vi "Batched Execution Engine.vi"() -> ()   [LabVIEW 2010]
uses:
  <vilib>/addons/database/NI_Database_API.lvlib
  <vilib>/addons/database/_DB Variant To Data/Database Variant To Data.xnode
  <vilib>/addons/database/Connection.llb/DB Tools Open Connec (String).vi
  <vilib>/xml/NI_XML.lvlib
  <vilib>/Utility/VariantDataType/VariantType.lvlib
  <vilib>/addons/database/Connection.llb/Conn Execute.vi
  <vilib>/addons/database/Recordset.llb/Rec Destroy - Connection.vi
  <vilib>/Utility/config.llb/NI_LVConfig.lvlib
  <vilib>/Utility/config.llb/Read Key (String).vi
panel:
  in  "Number of Parameters":i32
  out "Parameters Array Size":i32
  out "submit_time":timestamp
  out "exec_time":timestamp
  in  "Parameter out":T1(array[cluster])
  out "error in (no error)":errorcluster
  out "exp_id":i32
  out "Result: XML Footer":string
  out "Result: XML Header":string
  out "Control TAG":string
  out "Indicator TAG":string
  out "Experiment VI":string
  out "Database":string
  out "CSG 2":csg caption="CSG"
  out "CDB 2":cdb caption="CDB"
  out "CXT 2":cxt caption="CXT"
  out "U 65":u64 caption="U 64"
  out "U 33":u32 caption="U 32"
  out "U 17":u16 caption="U 16"
  out "I 9":i64 caption="I 8"
  out "I 65":i64 caption="I 64"
  out "EXT 2":ext caption="EXT"
  out "I16 2":i16
  out "FXP 2":fxp<+,1,1> caption="FXP"
  out "Single 2":sgl
  out "I 33":i32 caption="I 32"
  out "U 9":i32 caption="U 8"
  out "String 2":string caption="String"
  out "Double 2":dbl caption="Double"
  in  "Parameter in":cluster{"parameter":string, "datatype":string}[](array[cluster])
  out "XML-String-out":string
  in  "input array":variant[](array[variant])
  out "output array":variant[](array[variant])
  out "parse errors":string
  in  "Root in":string="/experimentSpecification/terminal/function/"
  in  "Write Status to Log file":bool
  out "XML-String-in":string
  in  "Stop":bool
  out "Status":string
  # "Parameter Tag"
  # "Parameter data type"
  # "Result Tag"
  # "Result Attribute"
  # "Settings"
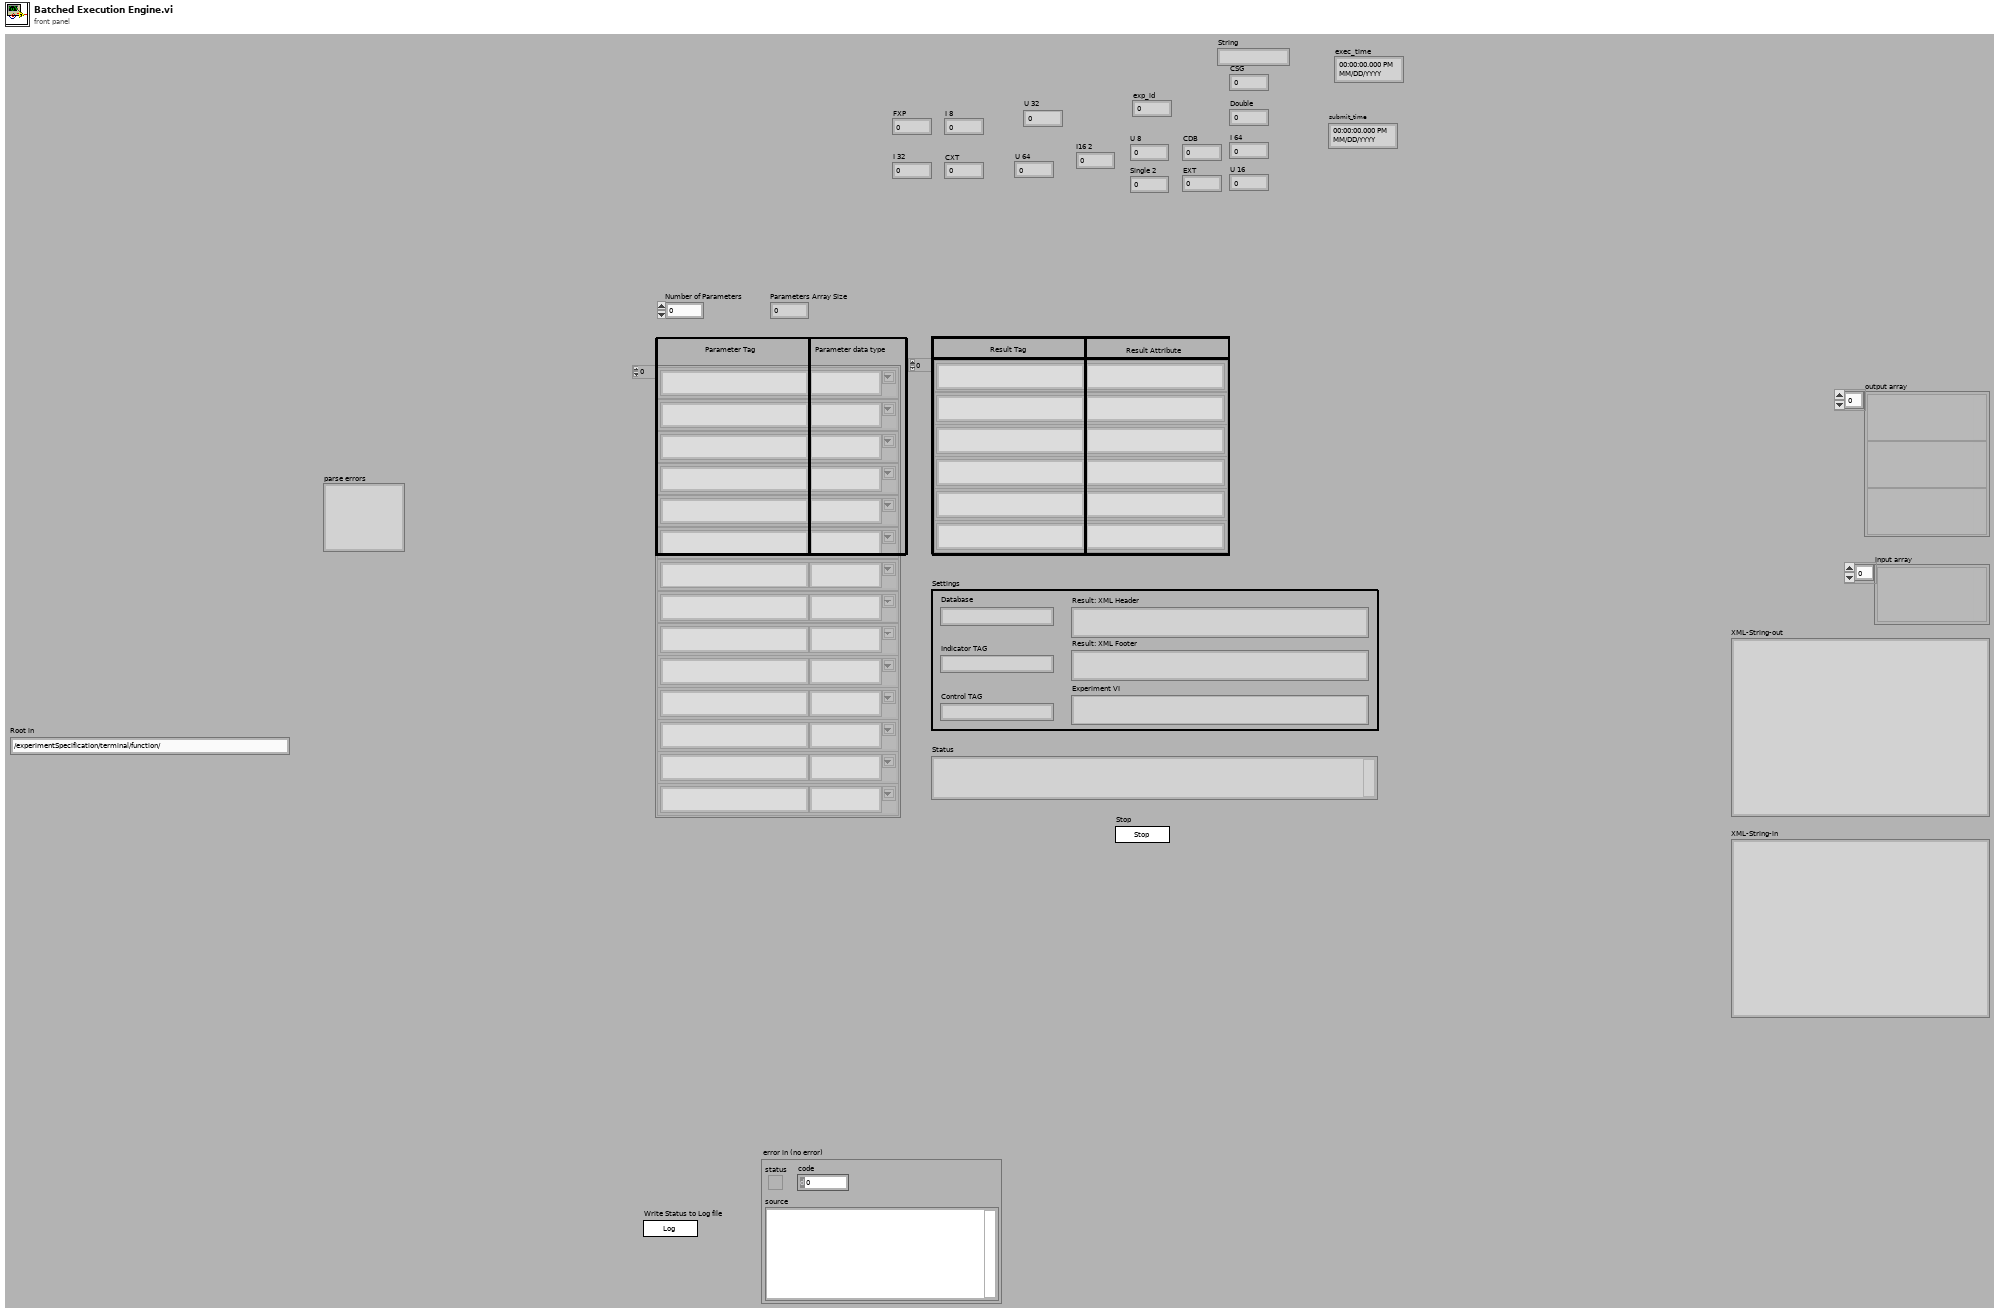
[diagram p1: front panel]
types:
  T1 = cluster{"parameter":string, "type info":string}[]
  T2 = enum16{"Search", "Parse", "Run", "Assemble", "Set", ""}
  T3 = typedef "NI_LVConfig.lvlib/Config Data RefNum.ctl" = refnum<k1>
  T4 = typedef "NI_Database_API.lvlib/Conn ObjectReference.ctl" = refnum<k1>
  T5 = typedef "NI_Database_API.lvlib/Rec ObjectReference.ctl" = refnum<k1>
  T6 = typedef "VariantType.lvlib/Type.ctl" = enum8{"Invalid Type", "Void", "I8", "I16", "I32", "I64", "U8", "U16", "U32", "U64", "Single Float", "Double Float", "Extended Float", "Single Complex", "Double Complex", "Extended Complex", "Enum U8", "Enum U16", "Enum U32", "Enum U64", "Single Float With Unit", "Double Float With Unit", "Extended Float With Unit", "Single Complex with Unit", "Double Complex with Unit", "Extended Complex with Unit", "Boolean", "String", "Path", "Picture", "Tag", "Array", "Cluster", "Variant", "LV Variant", "Waveform", "Timestamp", "Digital Waveform", "Digital Data", "ExpressData", "Refnum", "External Data", "VI", "Poly VI", "LabVIEW Class Instance", "Fixed Point"}
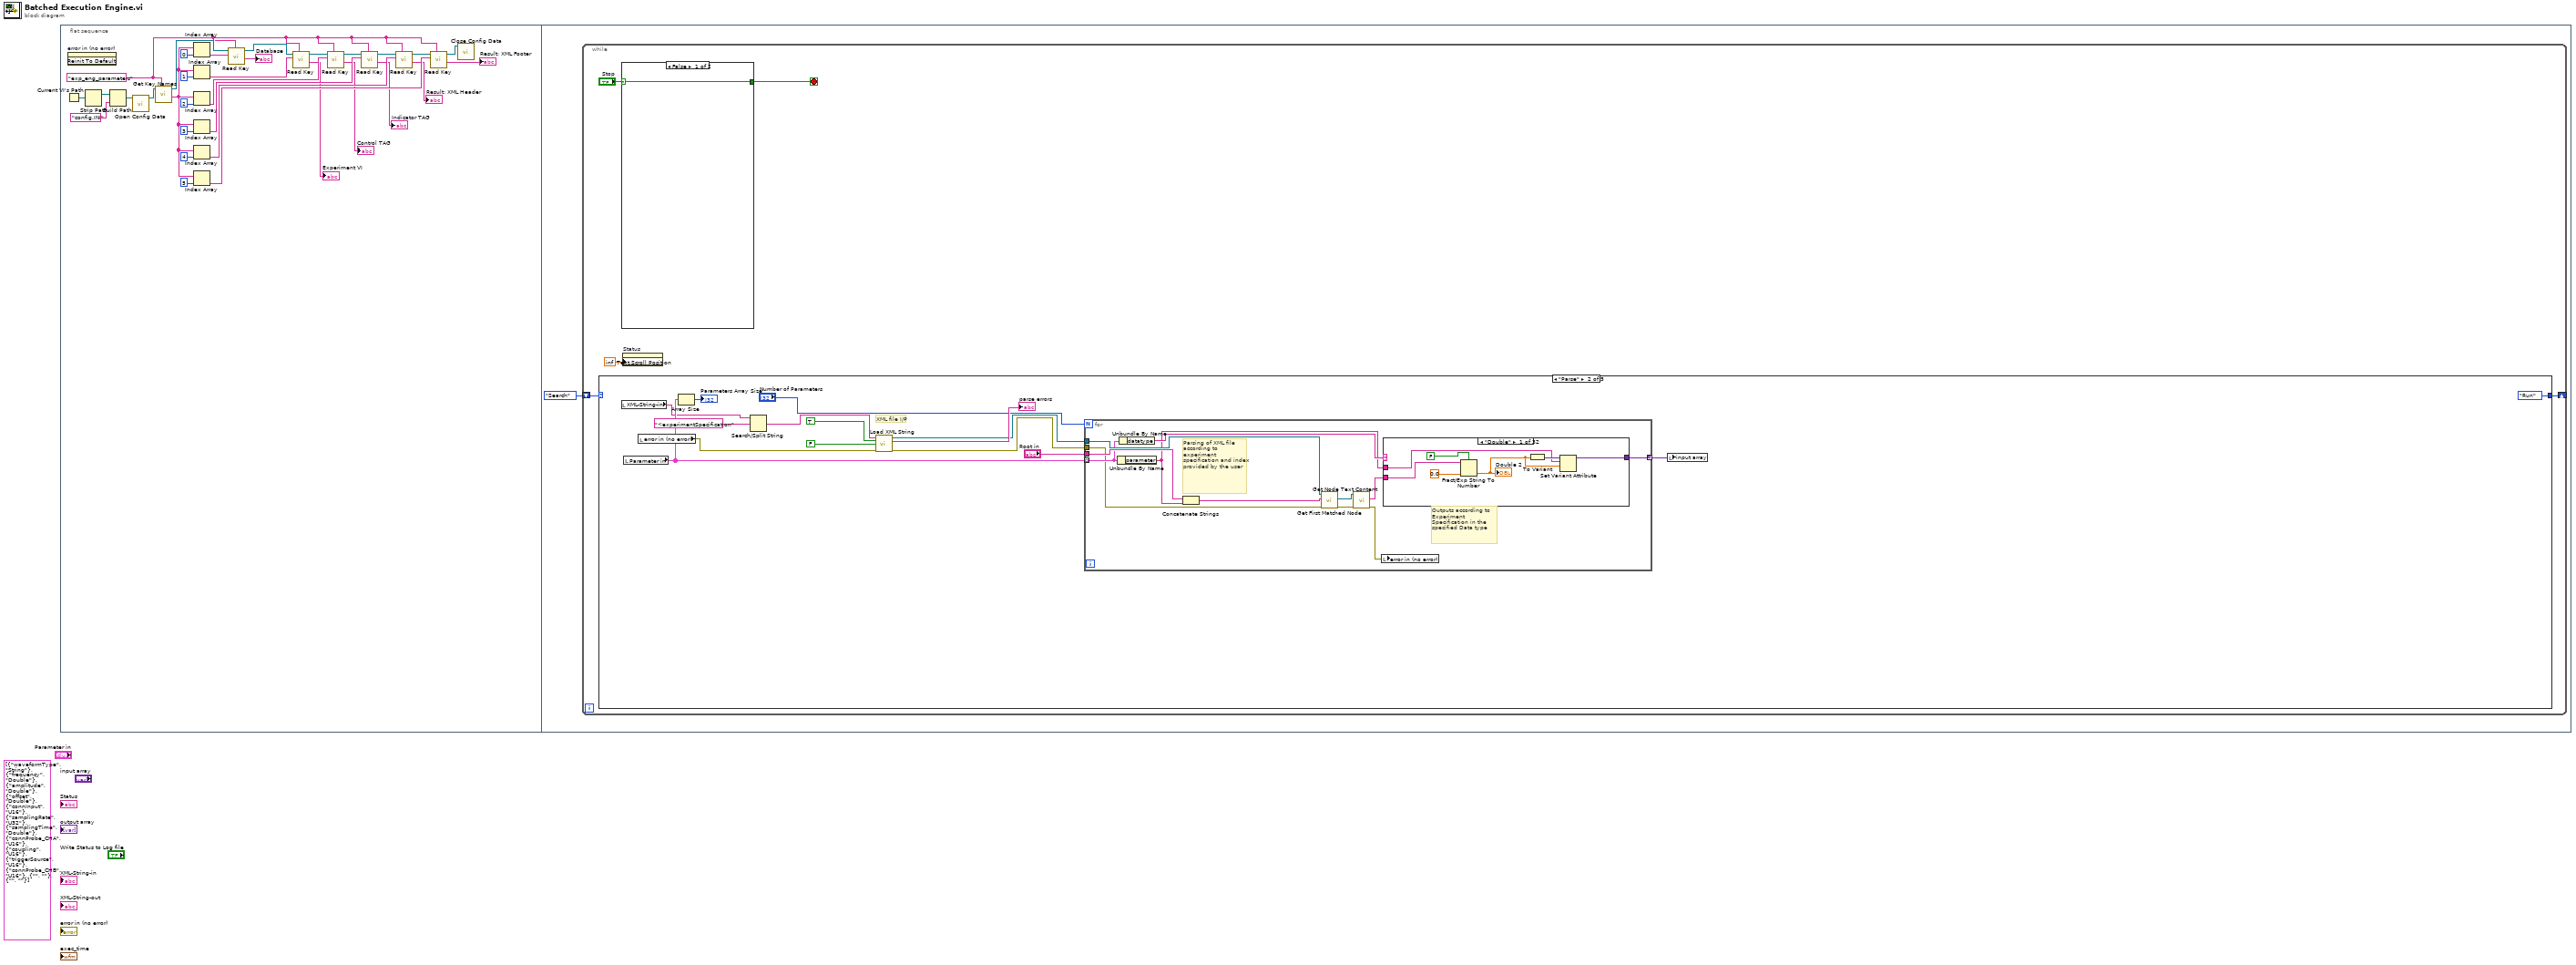
[diagram p0: block diagram]
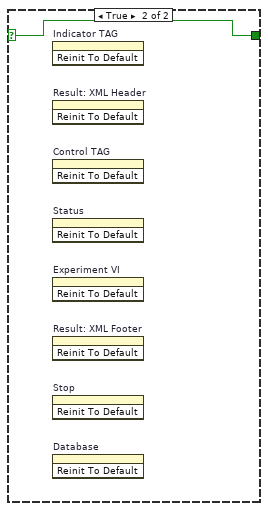
[diagram p2: hidden frame]
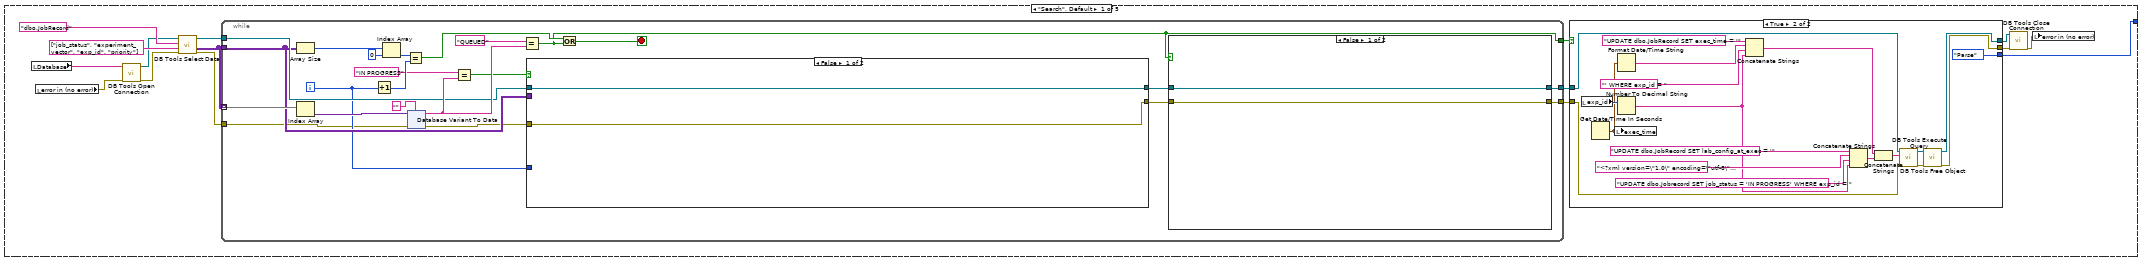
[diagram p3: hidden frame]
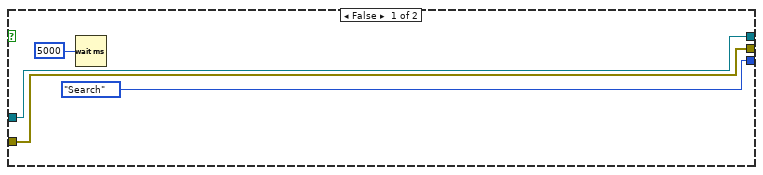
[diagram p4: hidden frame]
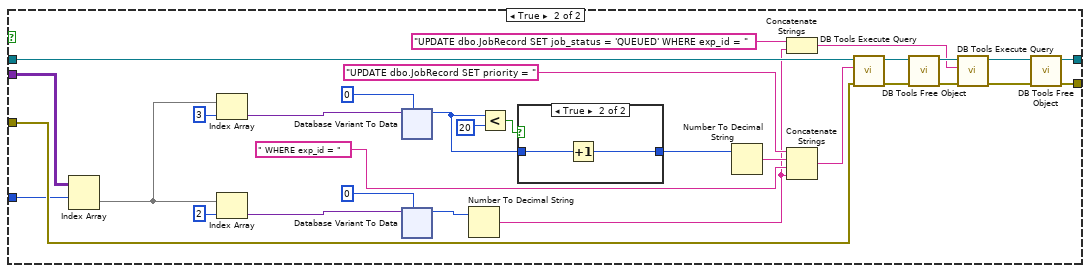
[diagram p5: hidden frame]
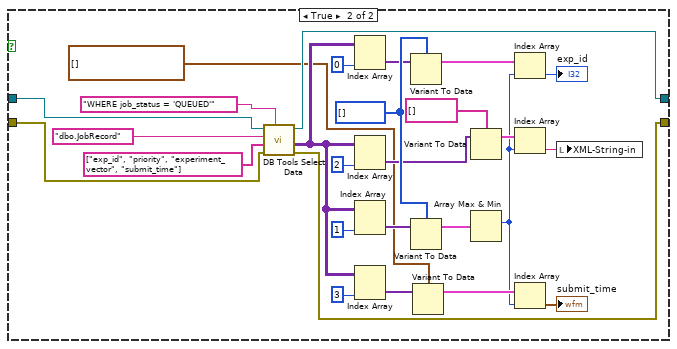
[diagram p7: hidden frame]
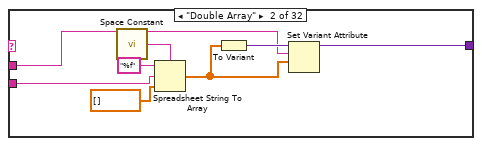
[diagram p8: hidden frame]
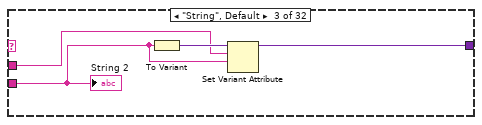
[diagram p9: hidden frame]
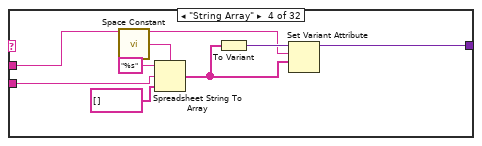
[diagram p10: hidden frame]
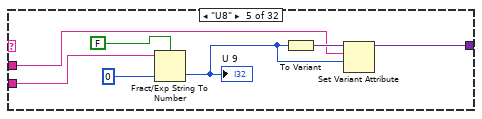
[diagram p11: hidden frame]
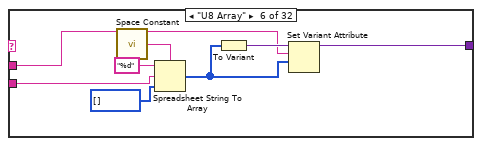
[diagram p12: hidden frame]
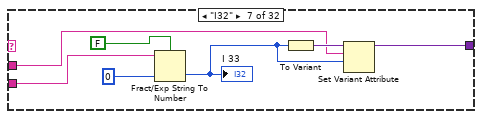
[diagram p13: hidden frame]
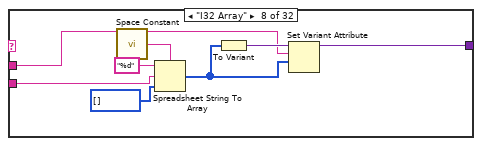
[diagram p14: hidden frame]
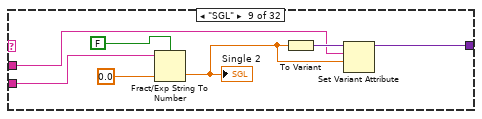
[diagram p15: hidden frame]
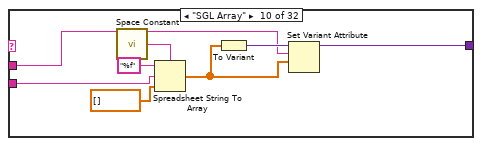
[diagram p16: hidden frame]
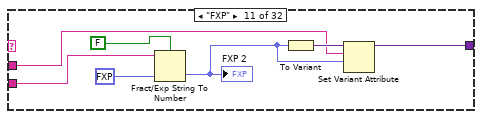
[diagram p17: hidden frame]
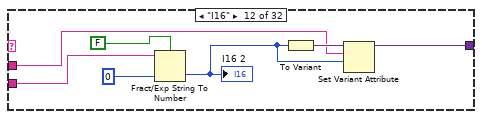
[diagram p18: hidden frame]
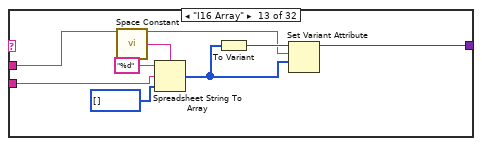
[diagram p19: hidden frame]
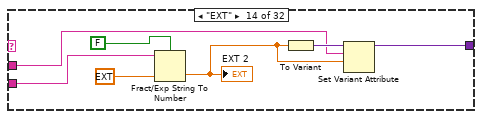
[diagram p20: hidden frame]
diagram:
  (unwired) cluster{"parameter":string, "datatype":string}[] [{"parameter"="waveformType", "datatype"="String"}, {"parameter"="frequency", "datatype"="Double"}, {"parameter"="amplitude", "datatype"="Double"}, {"parameter"="offset", "datatype"="Double"}, {"parameter"="connInput", "datatype"="U16"}, {"parameter"="samplingRate", "datatype"="U32"}, {"parameter"="samplingTime", "datatype"="Double"}, {"parameter"="connProbe_CHA", "datatype"="U16"}, {"parameter"="coupling", "datatype"="U16"}, {"parameter"="triggerSource", "datatype"="U16"}, {"parameter"="connProbe_CHB", "datatype"="U16"}, {"parameter"="", "datatype"=""}, {"parameter"="", "datatype"=""}] ("Parameter in")
  n1 = flat-sequence {
    frame #0 {
      w9 = "exp_eng_parameters" ("section")
      n2 = Current VI's Path() -> (path=w32:path)
      n3 = invoke on="error in (no error)" class="Clust (strict)" method="Reinit To Default"() -> ()  [unwired: 3 in, 3 out]
      n4 = Strip Path(path=w32) -> (stripped path=w31:path)  [unwired: 1 out]
      n5 = Build Path(base path=w31, name or relative path="config.INI") -> (appended path=w30:path)
      n6 = call <vilib>:"Open Config Data.vi"("configuration file path"=w30) -> ("refnum"=w28:T3)  [unwired: 8 in, 2 out]
      n7 = call <vilib>:"Get Key Names.vi"("section"=w9, "refnum"=w28) -> ("key names"=w11:string[], "refnum out"=w27:T3)  [unwired: 6 in, 2 out]
      n8 = Index Array(array=w11, index=0) -> (element=w25:string)
      n9 = Index Array(array=w11, index=1) -> (element=w23:string)
      n10 = Index Array(array=w11, index=2) -> (element=w19:string)
      n11 = Index Array(array=w11, index=3) -> (element=w16:string)
      n12 = Index Array(array=w11, index=4) -> (element=w14:string)
      n13 = Index Array(array=w11, index=5) -> (element=w10:string)
      n14 = call-poly <vilib>:"Read Key.vi"("section"=w9, "key"=w25, "refnum"=w27) -> ("value"=→"Database":string, "refnum out"=w22:T3)  [unwired: 5 in, 2 out]
      n15 = call-poly <vilib>:"Read Key.vi"("section"=w9, "key"=w23, "refnum"=w22) -> ("value"=→"Experiment VI":string, "refnum out"=w20:T3)  [unwired: 5 in, 2 out]
      n16 = call-poly <vilib>:"Read Key.vi"("section"=w9, "key"=w19, "refnum"=w20) -> ("value"=→"Control TAG":string, "refnum out"=w17:T3)  [unwired: 5 in, 2 out]
      n17 = call-poly <vilib>:"Read Key.vi"("section"=w9, "key"=w16, "refnum"=w17) -> ("value"=→"Indicator TAG":string, "refnum out"=w13:T3)  [unwired: 5 in, 2 out]
      n18 = call-poly <vilib>:"Read Key.vi"("section"=w9, "key"=w14, "refnum"=w13) -> ("value"=→"Result: XML Header":string, "refnum out"=w8:T3)  [unwired: 5 in, 2 out]
      n19 = call-poly <vilib>:"Read Key.vi"("section"=w9, "key"=w10, "refnum"=w8) -> ("value"=→"Result: XML Footer":string, "refnum out"=w7:T3)  [unwired: 5 in, 2 out]
      n20 = call <vilib>:"Close Config Data.vi"("refnum"=w7) -> ()  [unwired: 9 in, 2 out]
    }
    frame #1 {
      n21 = while {
        shift-right: [w37] -> _
        shift-left: T2."Search" -> [w38]
        stop <- w34 stop-if-true
        n22 = case shown="\"Parse\"" w38 {
          tunnel: [w52 T2."Run" T2."Assemble" T2."Set" T2."Search"] -> w37
          frame "Search", Default {
            n23 = local read "Database"() -> (w51:string)
            n24 = local read "error in (no error)"() -> (w47:errorcluster)
            n25 = call-poly <vilib>:"DB Tools Open Connection.vi"("error in (no error)"=w47, "connection information"=w51) -> ("error out"=w54:errorcluster, "connection reference"=w42:T4)  [unwired: 6 in]
            n26 = call <vilib>:"DB Tools Select Data.vi"("error in (no error)"=w54, "columns"=string[] ["job_status", "experiment_vector", "exp_id", "priority"], "table"="dbo.JobRecord", "connection reference"=w42) -> ("error out"=w46:errorcluster, "data"=w53:variant[][], "connection reference out"=w41:T4)  [unwired: 2 in]
            n27 = while {
              tunnel: w41 -> [w90]
              tunnel: [w94] -> w50
              tunnel: w53 -> [w99] mode=indexing
              tunnel: w53 -> [w88]
              tunnel: [w85] -> w43
              tunnel: w46 -> [w81]
              tunnel: [w82] -> w45
              i -> [w87]
              stop <- w84 stop-if-true
              n28 = Array Size(array=w88) -> (size(s)=w98:i32[])
              n29 = Index Array(array=w99) -> (element=w100:variant)  [unwired: 1 in]
              n30 = Increment(x=w87) -> (x+1=w95:i32)
              n31 = Index Array(array=w98, index=0) -> (element=w96:i32)
              n32 = Equal?(x=w96, y=w95) -> (x = y?=w86:bool)
              n33 = xnode "Database Variant To Data"("database variant"=w100, "error in"=w81, "type"="") -> ("data"=w93:string, "error out"=w80:errorcluster)
              n34 = Equal?(x="IN PROGRESS", y=w93) -> (x = y?=w91:bool)
              n35 = Equal?(x="QUEUED", y=w93) -> (x = y?=w85:bool)
              n36 = case shown="False" w91 {
                tunnel: w90 -> [w104 w124]
                tunnel: [w104 w120] -> w89
                tunnel: w88 -> [_ w135]
                tunnel: w87 -> [_ w105]
                tunnel: w80 -> [w103 w111]
                tunnel: [w103 w107] -> w83
                frame False {
                }
                frame True {
                  n37 = Index Array(array=w135, index (row)=w105) -> (element=w128:variant[])  [unwired: 1 in]
                  n38 = Index Array(array=w128, index=3) -> (element=w133:variant)
                  n39 = Index Array(array=w128, index=2) -> (element=w126:variant)
                  n40 = xnode "Database Variant To Data"("database variant"=w133, "type"=0 ("index")) -> ("data"=w129:i32)  [unwired: 1 in, 1 out]
                  n41 = xnode "Database Variant To Data"("database variant"=w126, "type"=0 ("index")) -> ("data"=w115:i32)  [unwired: 1 in, 1 out]
                  n42 = Number To Decimal String(number=w115) -> (decimal integer string=w112:string)  [unwired: 1 in]
                  n43 = Less?(x=w129, y=20) -> (x < y?=w130:bool)
                  n44 = case shown="True" w130 {
                    tunnel: w129 -> [w168 w170]
                    tunnel: [w168 w169] -> w118
                    frame False {
                    }
                    frame True {
                      n45 = Increment(x=w170) -> (x+1=w169:i32)
                    }
                  }
                  n46 = Number To Decimal String(number=w118) -> (decimal integer string=w117:string)  [unwired: 1 in]
                  n47 = Concatenate Strings("UPDATE dbo.JobRecord SET job_status = 'QUEUED' WHERE exp_id = " ("string"), w112) -> (w106:string)
                  n48 = Concatenate Strings("UPDATE dbo.JobRecord SET priority = " ("string"), w117, " WHERE exp_id = " ("string"), w112) -> (w114:string)
                  n49 = call-poly <vilib>:"DB Tools Execute Query.vi"("error in (no error)"=w111, "SQL query"=w114, "connection reference"=w124) -> ("error out"=w110:errorcluster, "recordset reference"=w123:T5)  [unwired: 5 in]
                  n50 = call-poly <vilib>:"DB Tools Free Object.vi"("error in (no error)"=w110, "recordset reference"=w123) -> ("error out"=w109:errorcluster, "connection reference"=w122:T4)  [unwired: 8 in]
                  n51 = call-poly <vilib>:"DB Tools Execute Query.vi"("error in (no error)"=w109, "SQL query"=w106, "connection reference"=w122) -> ("error out"=w108:errorcluster, "recordset reference"=w121:T5)  [unwired: 5 in]
                  n52 = call-poly <vilib>:"DB Tools Free Object.vi"("error in (no error)"=w108, "recordset reference"=w121) -> ("error out"=w107:errorcluster, "connection reference"=w120:T4)  [unwired: 8 in]
                }
              }
              n53 = Or(x=w86, y=w85) -> (x .or. y?=w84:bool)
              n54 = case shown="False" w85 {
                tunnel: w89 -> [w236 w254]
                tunnel: [w236 w253] -> w94
                tunnel: w83 -> [w235 w248]
                tunnel: [w235 w247] -> w82
                frame False {
                }
                frame True {
                  w261 = i32[] [] ("Array")
                  n55 = call <vilib>:"DB Tools Select Data.vi"("condition"="WHERE job_status = 'QUEUED'" ("optional clause"), "error in (no error)"=w248, "columns"=string[] ["exp_id", "priority", "experiment_vector", "submit_time"], "table"="dbo.JobRecord", "connection reference"=w254) -> ("error out"=w247:errorcluster, "data"=w243:variant[][], "connection reference out"=w253:T4)  [unwired: 1 in]
                  n56 = Index Array(array=w243, index (col)=0 ("disabled index (col)")) -> (element=w260:variant[])  [unwired: 1 in]
                  n57 = Index Array(array=w243, index (col)=2 ("index (row)")) -> (element=w251:variant[])  [unwired: 1 in]
                  n58 = Index Array(array=w243, index (col)=1 ("disabled index (col)")) -> (element=w258:variant[])  [unwired: 1 in]
                  n59 = Index Array(array=w243, index (col)=3 ("disabled index (col)")) -> (element=w241:variant[])  [unwired: 1 in]
                  n60 = Variant To Data(Variant=w260, type=w261) -> (data=w263:cluster{})  [unwired: 1 in, 1 out]
                  n61 = Variant To Data(Variant=w258, type=w261) -> (data=w262:cluster{})  [unwired: 1 in, 1 out]
                  n62 = Variant To Data(Variant=w241, type=timestamp[] [] ("Array")) -> (data=w239:cluster{})  [unwired: 1 in, 1 out]
                  n63 = Variant To Data(Variant=w251, type=string[] [] ("Array")) -> (data=w250:cluster{})  [unwired: 1 in, 1 out]
                  n64 = Array Max & Min(array=w262) -> (max index (indices)=w238:i32)  [unwired: 3 out]
                  n65 = Index Array(array=w263, index=w238) -> (element=→"exp_id":i32)
                  n66 = Index Array(array=w250, index=w238) -> (element=w249:string)
                  n67 = Index Array(array=w239, index=w238) -> (element=→"submit_time":timestamp)
                  n68 = local write "XML-String-in"(w249) -> ()
                }
              }
            }
            n69 = case shown="True" w43 {
              tunnel: [T2."Search" T2."Parse"] -> w52
              tunnel: [w60 w72] -> w49
              tunnel: w50 -> [w60 w78]
              tunnel: w45 -> [w59 w77]
              tunnel: [w59 w75] -> w48
              frame False {
                n70 = Wait (ms)(milliseconds to wait=u32 5000 ("millisecond multiple")) -> ()  [unwired: 1 out]
              }
              frame True {
                n71 = local read "exp_id"() -> (w74:i32)
                n72 = Get Date/Time In Seconds() -> (seconds since 1Jan1904=w61:timestamp)
                n73 = local write "exec_time"(w61) -> ()
                n74 = Format Date/Time String(seconds (now)=w61) -> (date/time string=w70:string)  [unwired: 2 in]
                n75 = Number To Decimal String(number=w74) -> (decimal integer string=w65:string)  [unwired: 1 in]
                n76 = Concatenate Strings("UPDATE dbo.JobRecord SET exec_time = '", w70, "' WHERE exp_id = ", w65) -> (w64:string)
                n77 = Concatenate Strings("UPDATE dbo.JobRecord SET lab_config_at_exec = '" ("string"), "<?xml version=\"1.0\" encoding=\"utf-8\" standalone=\"no\" ?><!DOCTYPE labConfiguration SYSTEM \"http://web.mit.edu/weblab/xml/labConfiguration.dtd\"><labConfiguration lab=\"MIT ELVIS Weblab\" specversion=\"0.1\">'" ("string"), "UPDATE dbo.Jobrecord SET job_status = 'IN PROGRESS' WHERE exp_id = " ("string"), w65) -> (w63:string)
                n78 = Concatenate Strings(w64, w63) -> (w62:string)
                n79 = call-poly <vilib>:"DB Tools Execute Query.vi"("error in (no error)"=w77, "SQL query"=w62, "connection reference"=w78) -> ("error out"=w76:errorcluster, "recordset reference"=w73:T5)  [unwired: 5 in]
                n80 = call-poly <vilib>:"DB Tools Free Object.vi"("error in (no error)"=w76, "recordset reference"=w73) -> ("error out"=w75:errorcluster, "connection reference"=w72:T4)  [unwired: 8 in]
              }
            }
            n81 = call <vilib>:"DB Tools Close Connection.vi"("error in (no error)"=w48, "connection reference"=w49) -> ("error out"=w44:errorcluster)  [unwired: 5 in]
            n82 = local write "error in (no error)"(w44) -> ()
          }
          frame "Parse" {
            # "XML file I/P"
            n83 = local read "XML-String-in"() -> (w268:string)
            n84 = local read "Parameter in"() -> (w271:cluster{"parameter":string, "datatype":string}[])
            n85 = local read "error in (no error)"() -> (w269:errorcluster)
            n86 = Array Size(array=w271) -> (size(s)=→"Parameters Array Size":i32)
            n87 = Search/Split String(string=w268, search string/char (-)="<experimentSpecification") -> (match + rest of string=w266:string)  [unwired: 1 in, 2 out]
            n88 = call <vilib>:"Load XML String.vi"("XML string"=w266, "process namespaces (False)"=TRUE, "process schema (False)"=FALSE, "error in (no error)"=w269) -> ("DOM document out"=w273:refnum<k20>, "parse errors"=→"parse errors":string, "error out"=w274:errorcluster)  [unwired: 9 out]
            n89 = for {
              N: "Number of Parameters" -> [_]
              tunnel: w273 -> [w290]
              tunnel: "Root in" -> [w287]
              tunnel: w271 -> [w285] mode=indexing
              tunnel: w274 -> [w284]
              tunnel: [w283] -> w270 mode=indexing
              # "Outputs according to Experiment Specification in the specified Data type"
              # "Parsing of XML file according to experiment specification and index provided by the user"
              n90 = Unbundle By Name(w285) -> ("parameter"=w280:string)
              n91 = Unbundle By Name(w285) -> ("datatype"=w282:string)
              n92 = Concatenate Strings(w287, w280) -> (w286:string)
              n93 = call <vilib>:"Get First Matched Node.vi"("error in (no error)"=w284, "XPath expression"=w286, "node in"=w290) -> ("error out"=w288:errorcluster, "node result"=w289:refnum<k20>)  [unwired: 6 in, 1 out]
              n94 = call <vilib>:"Get Node Text Content.vi"("error in (no error)"=w288, "node in"=w289) -> ("error out"=w279:errorcluster, "node text"=w281:string)  [unwired: 7 in, 1 out]
              n95 = local write "error in (no error)"(w279) -> ()
              n96 = case shown="\"Double\"" w282 {
                tunnel: w280 -> [w291 w299 w306 w310 w318 w325 w333 w341 w348 w356 w363 w370 w377 w385 w393 w400 w407 w415 w422 w430 w437 w445 w452 w460 w467 w475 w483 w491 w498 w505 w513 w520]
                tunnel: w281 -> [w292 w298 w307 w311 w319 w326 w334 w340 w349 w355 w364 w371 w378 w386 w392 w401 w408 w416 w423 w431 w438 w446 w453 w461 w468 w476 w482 w490 w497 w506 w512 w521]
                tunnel: [w294 w301 w308 w314 w321 w329 w336 w344 w351 w358 w366 w373 w381 w388 w395 w403 w411 w418 w426 w433 w441 w448 w456 w463 w471 w478 w485 w493 w500 w508 w515 w523] -> w283
                frame "Double" {
                  n97 = Fract/Exp String To Number(use system decimal point (T)=FALSE, string=w292, default (0 dbl)=0.0) -> (number=w293:dbl)  [unwired: 1 in, 1 out]
                  "Double 2" <- w293
                  n98 = To Variant(anything=w293) -> (Variant=w295:variant)
                  n99 = Set Variant Attribute(Variant=w295, name=w291, value=w293) -> (Variant out=w294:variant)  [unwired: 1 in, 2 out]
                }
                frame "Double Array" {
                  n100 = call <vilib>:"Space Constant.vi"() -> ("String"=w303:string)
                  n101 = Spreadsheet String To Array(delimiter (Tab)=w303, format string="%f", spreadsheet string=w298, array type (2D Dbl)=dbl[] [] ("Array")) -> (array=w300:dbl[])
                  n102 = To Variant(anything=w300) -> (Variant=w302:variant)
                  n103 = Set Variant Attribute(Variant=w302, name=w299, value=w300) -> (Variant out=w301:variant)  [unwired: 1 in, 2 out]
                }
                frame "String", Default {
                  n104 = To Variant(anything=w307) -> (Variant=w309:variant)
                  n105 = Set Variant Attribute(Variant=w309, name=w306, value=w307) -> (Variant out=w308:variant)  [unwired: 1 in, 2 out]
                  "String 2" <- w307
                }
                frame "String Array" {
                  n106 = call <vilib>:"Space Constant.vi"() -> ("String"=w316:string)
                  n107 = Spreadsheet String To Array(delimiter (Tab)=w316, format string="%s", spreadsheet string=w311, array type (2D Dbl)=string[] [] ("Array")) -> (array=w313:string[])
                  n108 = To Variant(anything=w313) -> (Variant=w315:variant)
                  n109 = Set Variant Attribute(Variant=w315, name=w310, value=w313) -> (Variant out=w314:variant)  [unwired: 1 in, 2 out]
                }
                frame "U8" {
                  n110 = Fract/Exp String To Number(use system decimal point (T)=FALSE, string=w319, default (0 dbl)=u8 0) -> (number=w320:u8)  [unwired: 1 in, 1 out]
                  "U 9" <- w320
                  n111 = To Variant(anything=w320) -> (Variant=w322:variant)
                  n112 = Set Variant Attribute(Variant=w322, name=w318, value=w320) -> (Variant out=w321:variant)  [unwired: 1 in, 2 out]
                }
                frame "U8 Array" {
                  n113 = call <vilib>:"Space Constant.vi"() -> ("String"=w331:string)
                  n114 = Spreadsheet String To Array(delimiter (Tab)=w331, format string="%d", spreadsheet string=w326, array type (2D Dbl)=u8[] [] ("Array")) -> (array=w327:u8[])
                  n115 = To Variant(anything=w327) -> (Variant=w330:variant)
                  n116 = Set Variant Attribute(Variant=w330, name=w325, value=w327) -> (Variant out=w329:variant)  [unwired: 1 in, 2 out]
                }
                frame "I32" {
                  n117 = Fract/Exp String To Number(use system decimal point (T)=FALSE, string=w334, default (0 dbl)=0) -> (number=w335:i32)  [unwired: 1 in, 1 out]
                  "I 33" <- w335
                  n118 = To Variant(anything=w335) -> (Variant=w337:variant)
                  n119 = Set Variant Attribute(Variant=w337, name=w333, value=w335) -> (Variant out=w336:variant)  [unwired: 1 in, 2 out]
                }
                frame "I32 Array" {
                  n120 = call <vilib>:"Space Constant.vi"() -> ("String"=w346:string)
                  n121 = Spreadsheet String To Array(delimiter (Tab)=w346, format string="%d", spreadsheet string=w340, array type (2D Dbl)=i32[] [] ("Array")) -> (array=w342:i32[])
                  n122 = To Variant(anything=w342) -> (Variant=w345:variant)
                  n123 = Set Variant Attribute(Variant=w345, name=w341, value=w342) -> (Variant out=w344:variant)  [unwired: 1 in, 2 out]
                }
                frame "SGL" {
                  n124 = Fract/Exp String To Number(use system decimal point (T)=FALSE, string=w349, default (0 dbl)=sgl 0.0) -> (number=w350:sgl)  [unwired: 1 in, 1 out]
                  "Single 2" <- w350
                  n125 = To Variant(anything=w350) -> (Variant=w352:variant)
                  n126 = Set Variant Attribute(Variant=w352, name=w348, value=w350) -> (Variant out=w351:variant)  [unwired: 1 in, 2 out]
                }
                frame "SGL Array" {
                  n127 = call <vilib>:"Space Constant.vi"() -> ("String"=w360:string)
                  n128 = Spreadsheet String To Array(delimiter (Tab)=w360, format string="%f", spreadsheet string=w355, array type (2D Dbl)=sgl[] [] ("Array")) -> (array=w357:sgl[])
                  n129 = To Variant(anything=w357) -> (Variant=w359:variant)
                  n130 = Set Variant Attribute(Variant=w359, name=w356, value=w357) -> (Variant out=w358:variant)  [unwired: 1 in, 2 out]
                }
                frame "FXP" {
                  n131 = Fract/Exp String To Number(use system decimal point (T)=FALSE, string=w364, default (0 dbl)=fxp<+,1,1> 0.0) -> (number=w365:fxp<+,1,1>)  [unwired: 1 in, 1 out]
                  "FXP 2" <- w365
                  n132 = To Variant(anything=w365) -> (Variant=w367:variant)
                  n133 = Set Variant Attribute(Variant=w367, name=w363, value=w365) -> (Variant out=w366:variant)  [unwired: 1 in, 2 out]
                }
                frame "I16" {
                  n134 = Fract/Exp String To Number(use system decimal point (T)=FALSE, string=w371, default (0 dbl)=i16 0 ("I16")) -> (number=w374:i16)  [unwired: 1 in, 1 out]
                  "I16 2" <- w374
                  n135 = To Variant(anything=w374) -> (Variant=w375:variant)
                  n136 = Set Variant Attribute(Variant=w375, name=w370, value=w374) -> (Variant out=w373:variant)  [unwired: 1 in, 2 out]
                }
                frame "I16 Array" {
                  n137 = call <vilib>:"Space Constant.vi"() -> ("String"=w383:string)
                  n138 = Spreadsheet String To Array(delimiter (Tab)=w383, format string="%d", spreadsheet string=w378, array type (2D Dbl)=i16[] [] ("Array")) -> (array=w379:i16[])
                  n139 = To Variant(anything=w379) -> (Variant=w382:variant)
                  n140 = Set Variant Attribute(Variant=w382, name=w377, value=w379) -> (Variant out=w381:variant)  [unwired: 1 in, 2 out]
                }
                frame "EXT" {
                  n141 = Fract/Exp String To Number(use system decimal point (T)=FALSE, string=w386, default (0 dbl)=ext 0.0) -> (number=w387:ext)  [unwired: 1 in, 1 out]
                  "EXT 2" <- w387
                  n142 = To Variant(anything=w387) -> (Variant=w389:variant)
                  n143 = Set Variant Attribute(Variant=w389, name=w385, value=w387) -> (Variant out=w388:variant)  [unwired: 1 in, 2 out]
                }
                frame "EXT Array" {
                  n144 = call <vilib>:"Space Constant.vi"() -> ("String"=w397:string)
                  n145 = Spreadsheet String To Array(delimiter (Tab)=w397, format string="%f", spreadsheet string=w392, array type (2D Dbl)=ext[] [] ("Array")) -> (array=w394:ext[])
                  n146 = To Variant(anything=w394) -> (Variant=w396:variant)
                  n147 = Set Variant Attribute(Variant=w396, name=w393, value=w394) -> (Variant out=w395:variant)  [unwired: 1 in, 2 out]
                }
                frame "I64" {
                  n148 = Fract/Exp String To Number(use system decimal point (T)=FALSE, string=w401, default (0 dbl)=i64 0) -> (number=w402:i64)  [unwired: 1 in, 1 out]
                  "I 65" <- w402
                  n149 = To Variant(anything=w402) -> (Variant=w404:variant)
                  n150 = Set Variant Attribute(Variant=w404, name=w400, value=w402) -> (Variant out=w403:variant)  [unwired: 1 in, 2 out]
                }
                frame "I64 Array" {
                  n151 = call <vilib>:"Space Constant.vi"() -> ("String"=w413:string)
                  n152 = Spreadsheet String To Array(delimiter (Tab)=w413, format string="%d", spreadsheet string=w408, array type (2D Dbl)=i64[] [] ("Array")) -> (array=w409:i64[])
                  n153 = To Variant(anything=w409) -> (Variant=w412:variant)
                  n154 = Set Variant Attribute(Variant=w412, name=w407, value=w409) -> (Variant out=w411:variant)  [unwired: 1 in, 2 out]
                }
                frame "I8" {
                  n155 = Fract/Exp String To Number(use system decimal point (T)=FALSE, string=w416, default (0 dbl)=i8 0) -> (number=w417:i8)  [unwired: 1 in, 1 out]
                  "I 9" <- w417
                  n156 = To Variant(anything=w417) -> (Variant=w419:variant)
                  n157 = Set Variant Attribute(Variant=w419, name=w415, value=w417) -> (Variant out=w418:variant)  [unwired: 1 in, 2 out]
                }
                frame "I8 Array" {
                  n158 = call <vilib>:"Space Constant.vi"() -> ("String"=w428:string)
                  n159 = Spreadsheet String To Array(delimiter (Tab)=w428, format string="%d", spreadsheet string=w423, array type (2D Dbl)=i8[] [] ("Array")) -> (array=w424:i8[])
                  n160 = To Variant(anything=w424) -> (Variant=w427:variant)
                  n161 = Set Variant Attribute(Variant=w427, name=w422, value=w424) -> (Variant out=w426:variant)  [unwired: 1 in, 2 out]
                }
                frame "U16" {
                  n162 = Fract/Exp String To Number(use system decimal point (T)=FALSE, string=w431, default (0 dbl)=u16 0) -> (number=w432:u16)  [unwired: 1 in, 1 out]
                  "U 17" <- w432
                  n163 = To Variant(anything=w432) -> (Variant=w434:variant)
                  n164 = Set Variant Attribute(Variant=w434, name=w430, value=w432) -> (Variant out=w433:variant)  [unwired: 1 in, 2 out]
                }
                frame "U16 Array" {
                  n165 = call <vilib>:"Space Constant.vi"() -> ("String"=w443:string)
                  n166 = Spreadsheet String To Array(delimiter (Tab)=w443, format string="%d", spreadsheet string=w438, array type (2D Dbl)=u16[] [] ("Array")) -> (array=w439:u16[])
                  n167 = To Variant(anything=w439) -> (Variant=w442:variant)
                  n168 = Set Variant Attribute(Variant=w442, name=w437, value=w439) -> (Variant out=w441:variant)  [unwired: 1 in, 2 out]
                }
                frame "U32" {
                  n169 = Fract/Exp String To Number(use system decimal point (T)=FALSE, string=w446, default (0 dbl)=u32 0) -> (number=w447:u32)  [unwired: 1 in, 1 out]
                  "U 33" <- w447
                  n170 = To Variant(anything=w447) -> (Variant=w449:variant)
                  n171 = Set Variant Attribute(Variant=w449, name=w445, value=w447) -> (Variant out=w448:variant)  [unwired: 1 in, 2 out]
                }
                frame "U32 Array" {
                  n172 = call <vilib>:"Space Constant.vi"() -> ("String"=w458:string)
                  n173 = Spreadsheet String To Array(delimiter (Tab)=w458, format string="%d", spreadsheet string=w453, array type (2D Dbl)=u32[] [] ("Array")) -> (array=w454:u32[])
                  n174 = To Variant(anything=w454) -> (Variant=w457:variant)
                  n175 = Set Variant Attribute(Variant=w457, name=w452, value=w454) -> (Variant out=w456:variant)  [unwired: 1 in, 2 out]
                }
                frame "U64" {
                  n176 = Fract/Exp String To Number(use system decimal point (T)=FALSE, string=w461, default (0 dbl)=u64 0) -> (number=w462:u64)  [unwired: 1 in, 1 out]
                  "U 65" <- w462
                  n177 = To Variant(anything=w462) -> (Variant=w464:variant)
                  n178 = Set Variant Attribute(Variant=w464, name=w460, value=w462) -> (Variant out=w463:variant)  [unwired: 1 in, 2 out]
                }
                frame "U64 Array" {
                  n179 = call <vilib>:"Space Constant.vi"() -> ("String"=w473:string)
                  n180 = Spreadsheet String To Array(delimiter (Tab)=w473, format string="%d", spreadsheet string=w468, array type (2D Dbl)=u64[] [] ("Array")) -> (array=w469:u64[])
                  n181 = To Variant(anything=w469) -> (Variant=w472:variant)
                  n182 = Set Variant Attribute(Variant=w472, name=w467, value=w469) -> (Variant out=w471:variant)  [unwired: 1 in, 2 out]
                }
                frame "CXT" {
                  n183 = Scan From String(format string="%f", input string=w476, default 1=cxt 0.0+0.0i ("number 3")) -> (output 1=w477:cxt)  [unwired: 2 in, 3 out]
                  "CXT 2" <- w477
                  n184 = To Variant(anything=w477) -> (Variant=w479:variant)
                  n185 = Set Variant Attribute(Variant=w479, name=w475, value=w477) -> (Variant out=w478:variant)  [unwired: 1 in, 2 out]
                }
                frame "CXT Array" {
                  n186 = call <vilib>:"Space Constant.vi"() -> ("String"=w487:string)
                  n187 = Spreadsheet String To Array(delimiter (Tab)=w487, format string="%f", spreadsheet string=w482, array type (2D Dbl)=cxt[] [] ("Array")) -> (array=w484:cxt[])
                  n188 = To Variant(anything=w484) -> (Variant=w486:variant)
                  n189 = Set Variant Attribute(Variant=w486, name=w483, value=w484) -> (Variant out=w485:variant)  [unwired: 1 in, 2 out]
                }
                frame "CDB" {
                  n190 = Scan From String(format string="%f", input string=w490, default 1=cdb 0.0+0.0i ("number 3")) -> (output 1=w492:cdb)  [unwired: 2 in, 3 out]
                  "CDB 2" <- w492
                  n191 = To Variant(anything=w492) -> (Variant=w494:variant)
                  n192 = Set Variant Attribute(Variant=w494, name=w491, value=w492) -> (Variant out=w493:variant)  [unwired: 1 in, 2 out]
                }
                frame "CDB Array" {
                  n193 = call <vilib>:"Space Constant.vi"() -> ("String"=w502:string)
                  n194 = Spreadsheet String To Array(delimiter (Tab)=w502, format string="%f", spreadsheet string=w497, array type (2D Dbl)=cdb[] [] ("Array")) -> (array=w499:cdb[])
                  n195 = To Variant(anything=w499) -> (Variant=w501:variant)
                  n196 = Set Variant Attribute(Variant=w501, name=w498, value=w499) -> (Variant out=w500:variant)  [unwired: 1 in, 2 out]
                }
                frame "CSG" {
                  n197 = Scan From String(format string="%f", input string=w506, default 1=csg 0.0+0.0i ("number 3")) -> (output 1=w507:csg)  [unwired: 2 in, 3 out]
                  "CSG 2" <- w507
                  n198 = To Variant(anything=w507) -> (Variant=w509:variant)
                  n199 = Set Variant Attribute(Variant=w509, name=w505, value=w507) -> (Variant out=w508:variant)  [unwired: 1 in, 2 out]
                }
                frame "CSG Array" {
                  n200 = call <vilib>:"Space Constant.vi"() -> ("String"=w517:string)
                  n201 = Spreadsheet String To Array(delimiter (Tab)=w517, format string="%f", spreadsheet string=w512, array type (2D Dbl)=csg[] [] ("Array")) -> (array=w514:csg[])
                  n202 = To Variant(anything=w514) -> (Variant=w516:variant)
                  n203 = Set Variant Attribute(Variant=w516, name=w513, value=w514) -> (Variant out=w515:variant)  [unwired: 1 in, 2 out]
                }
                frame "Boolean" {
                  n204 = case shown="\"False\", Default" w521 {
                    tunnel: [FALSE TRUE TRUE FALSE TRUE FALSE TRUE FALSE] -> w522
                    frame "False", Default {
                    }
                    frame "True" {
                    }
                    frame "TRUE" {
                    }
                    frame "FALSE" {
                    }
                    frame "1" {
                    }
                    frame "0" {
                    }
                    frame "true" {
                    }
                    frame "false" {
                    }
                  }
                  n205 = To Variant(anything=w522) -> (Variant=w524:variant)
                  n206 = Set Variant Attribute(Variant=w524, name=w520, value=w522) -> (Variant out=w523:variant)  [unwired: 1 in, 2 out]
                }
              }
            }
            n207 = local write "input array"(w270) -> ()
          }
          frame "Run" {
            n208 = local read "Experiment VI"() -> (w544:string)
            n209 = local read "Indicator TAG"() -> (w547:string)
            n210 = local read "Control TAG"() -> (w545:string)
            n211 = local read "input array"() -> (w542:variant[])
            n212 = local read "error in (no error)"() -> (w539:errorcluster)
            n213 = String To Path(string=w544) -> (path=w543:path)
            n214 = Open VI Reference(vi path=w543, error in (no error)=w539) -> (vi reference=w551:refnum<vi>, error out=w538:errorcluster)  [unwired: 4 in]
            n215 = invoke class="VI" method="Ctrl Val.Set"(reference=w551, error in=w538, "Control Name"=w545, "Value"=w542) -> (reference out=w546:refnum<vi>, error out=w537:errorcluster)  [unwired: 1 in, 3 out]
            n216 = invoke class="VI" method="Run VI"(reference=w546, error in=w537) -> (reference out=w550:refnum<vi>, error out=w536:errorcluster)  [unwired: 3 in, 3 out]
            n217 = invoke class="VI" method="Ctrl Val.Get"(reference=w550, error in=w536, "Control Name"=w547) -> (reference out=w548:refnum<vi>, error out=w535:errorcluster, "Get Control Value Variant"=w549:variant)  [unwired: 1 in, 1 out]
            n218 = Close Reference(reference=w548, error in (no error)=w535) -> (error out=w534:errorcluster)
            n219 = Variant To Data(error in=w534, Variant=w549, type=variant[] [variant(variant[] [variant(dbl[] array[3004 elements])])] ("output array")) -> (error out=w533:errorcluster, data=w540:cluster{})
            n220 = local write "output array"(w540) -> ()
            n221 = local write "error in (no error)"(w533) -> ()
          }
          frame "Assemble" {
            n222 = local read "output array"() -> (w556:variant[])
            n223 = local read "Result: XML Header"() -> (w555:string)
            n224 = local read "Result: XML Footer"() -> (w554:string)
            n225 = Array Size(array="Parameter out") -> (size(s)=w559:i32)
            n226 = for {
              N: w559 -> [_]
              tunnel: w556 -> [w564] mode=indexing
              tunnel: "Parameter out" -> [w562] mode=indexing
              tunnel: [w566] -> w557 mode=indexing
              n227 = call <vilib>:"GetTypeInfo.vi"("Variant"=w564) -> ("Type Enum"=w563:T6)  [unwired: 6 in, 4 out]
              n228 = Unbundle By Name(w562) -> ("parameter"=w565:string)
              n229 = Unbundle By Name(w562) -> ("type info"=w561:string)
              n230 = case shown="\"I8\"" w563 {
                tunnel: w565 -> [w568 w592 w617 w640 w665 w688 w712 w736 w760 w785 w810 w835 w859 w883 w907 w932 w1200 w1220]
                tunnel: [w567 w591 w615 w639 w664 w687 w711 w735 w759 w784 w809 w834 w858 w882 w906 w936 w1196 w1219] -> w566
                tunnel: w564 -> [w573 w597 w621 w645 w669 w693 w717 w741 w767 w792 w817 w840 w864 w888 w912 w937 w1202 w1228]
                tunnel: w561 -> [w570 w594 w618 w642 w663 w690 w714 w738 w762 w787 w812 w837 w861 w885 w909 w931 w1198 w1222]
                frame "I8" {
                  n231 = Get Variant Attribute(Variant=w573, name=w568) -> (duplicate Variant=w574:variant)  [unwired: 2 in, 3 out]
                  n232 = Equal?(x=w570, y="") -> (x = y?=w572:bool)
                  n233 = Variant To Data(Variant=w574, type=i8 0) -> (data=w576:cluster{})  [unwired: 1 in, 1 out]
                  n234 = Number To Decimal String(number=w576) -> (decimal integer string=w569:string)  [unwired: 1 in]
                  n235 = case shown="True" w572 {
                    tunnel: w568 -> [w580 w585]
                    tunnel: w570 -> [w577 _]
                    tunnel: w569 -> [w579 w588]
                    tunnel: [w578 w589] -> w567
                    frame False {
                      w583 = ">" ("string")
                      n236 = call <vilib>:"Space Constant.vi"() -> ("String"=w584:string)
                      n237 = Concatenate Strings("<" ("string"), w580, w584, w577, w583, w579, "</" ("string"), w580, w583) -> (w578:string)
                    }
                    frame True {
                      w586 = ">" ("string")
                      n238 = Concatenate Strings("<" ("string"), w585, w586, w588, "</" ("string"), w585, w586) -> (w589:string)
                    }
                  }
                }
                frame "I16" {
                  n239 = Get Variant Attribute(Variant=w597, name=w592) -> (duplicate Variant=w599:variant)  [unwired: 2 in, 3 out]
                  n240 = Equal?(x=w594, y="") -> (x = y?=w596:bool)
                  n241 = Variant To Data(Variant=w599, type=i16 0 ("I16")) -> (data=w600:cluster{})  [unwired: 1 in, 1 out]
                  n242 = Number To Decimal String(number=w600) -> (decimal integer string=w593:string)  [unwired: 1 in]
                  n243 = case shown="True" w596 {
                    tunnel: w592 -> [w604 w609]
                    tunnel: w594 -> [w601 _]
                    tunnel: w593 -> [w603 w612]
                    tunnel: [w602 w613] -> w591
                    frame False {
                      w607 = ">" ("string")
                      n244 = call <vilib>:"Space Constant.vi"() -> ("String"=w608:string)
                      n245 = Concatenate Strings("<" ("string"), w604, w608, w601, w607, w603, "</" ("string"), w604, w607) -> (w602:string)
                    }
                    frame True {
                      w610 = ">" ("string")
                      n246 = Concatenate Strings("<" ("string"), w609, w610, w612, "</" ("string"), w609, w610) -> (w613:string)
                    }
                  }
                }
                frame "I32" {
                  n247 = Get Variant Attribute(Variant=w621, name=w617) -> (duplicate Variant=w622:variant)  [unwired: 2 in, 3 out]
                  n248 = Equal?(x=w618, y="") -> (x = y?=w620:bool)
                  n249 = Variant To Data(Variant=w622, type=i16 0 ("precision (6)")) -> (data=w624:cluster{})  [unwired: 1 in, 1 out]
                  n250 = Number To Decimal String(number=w624) -> (decimal integer string=w616:string)  [unwired: 1 in]
                  n251 = case shown="True" w620 {
                    tunnel: w617 -> [w628 w633]
                    tunnel: w618 -> [w625 _]
                    tunnel: w616 -> [w627 w636]
                    tunnel: [w626 w637] -> w615
                    frame False {
                      w631 = ">" ("string")
                      n252 = call <vilib>:"Space Constant.vi"() -> ("String"=w632:string)
                      n253 = Concatenate Strings("<" ("string"), w628, w632, w625, w631, w627, "</" ("string"), w628, w631) -> (w626:string)
                    }
                    frame True {
                      w634 = ">" ("string")
                      n254 = Concatenate Strings("<" ("string"), w633, w634, w636, "</" ("string"), w633, w634) -> (w637:string)
                    }
                  }
                }
                frame "I64" {
                  n255 = Get Variant Attribute(Variant=w645, name=w640) -> (duplicate Variant=w646:variant)  [unwired: 2 in, 3 out]
                  n256 = Equal?(x=w642, y="") -> (x = y?=w644:bool)
                  n257 = Variant To Data(Variant=w646, type=i64 0) -> (data=w648:cluster{})  [unwired: 1 in, 1 out]
                  n258 = Number To Decimal String(number=w648) -> (decimal integer string=w641:string)  [unwired: 1 in]
                  n259 = case shown="True" w644 {
                    tunnel: w640 -> [w652 w657]
                    tunnel: w642 -> [w649 _]
                    tunnel: w641 -> [w651 w660]
                    tunnel: [w650 w661] -> w639
                    frame False {
                      w655 = ">" ("string")
                      n260 = call <vilib>:"Space Constant.vi"() -> ("String"=w656:string)
                      n261 = Concatenate Strings("<" ("string"), w652, w656, w649, w655, w651, "</" ("string"), w652, w655) -> (w650:string)
                    }
                    frame True {
                      w658 = ">" ("string")
                      n262 = Concatenate Strings("<" ("string"), w657, w658, w660, "</" ("string"), w657, w658) -> (w661:string)
                    }
                  }
                }
                frame "U8" {
                  n263 = Get Variant Attribute(Variant=w669, name=w665) -> (duplicate Variant=w670:variant)  [unwired: 2 in, 3 out]
                  n264 = Equal?(x=w663, y="") -> (x = y?=w668:bool)
                  n265 = Variant To Data(Variant=w670, type=u8 0) -> (data=w672:cluster{})  [unwired: 1 in, 1 out]
                  n266 = Number To Decimal String(number=w672) -> (decimal integer string=w666:string)  [unwired: 1 in]
                  n267 = case shown="True" w668 {
                    tunnel: w665 -> [w676 w681]
                    tunnel: w663 -> [w673 _]
                    tunnel: w666 -> [w675 w684]
                    tunnel: [w674 w685] -> w664
                    frame False {
                      w679 = ">" ("string")
                      n268 = call <vilib>:"Space Constant.vi"() -> ("String"=w680:string)
                      n269 = Concatenate Strings("<" ("string"), w676, w680, w673, w679, w675, "</" ("string"), w676, w679) -> (w674:string)
                    }
                    frame True {
                      w682 = ">" ("string")
                      n270 = Concatenate Strings("<" ("string"), w681, w682, w684, "</" ("string"), w681, w682) -> (w685:string)
                    }
                  }
                }
                frame "U16" {
                  n271 = Get Variant Attribute(Variant=w693, name=w688) -> (duplicate Variant=w694:variant)  [unwired: 2 in, 3 out]
                  n272 = Equal?(x=w690, y="") -> (x = y?=w692:bool)
                  n273 = Variant To Data(Variant=w694, type=u16 0) -> (data=w696:cluster{})  [unwired: 1 in, 1 out]
                  n274 = Number To Decimal String(number=w696) -> (decimal integer string=w689:string)  [unwired: 1 in]
                  n275 = case shown="True" w692 {
                    tunnel: w688 -> [w700 w705]
                    tunnel: w690 -> [w697 _]
                    tunnel: w689 -> [w699 w708]
                    tunnel: [w698 w709] -> w687
                    frame False {
                      w703 = ">" ("string")
                      n276 = call <vilib>:"Space Constant.vi"() -> ("String"=w704:string)
                      n277 = Concatenate Strings("<" ("string"), w700, w704, w697, w703, w699, "</" ("string"), w700, w703) -> (w698:string)
                    }
                    frame True {
                      w706 = ">" ("string")
                      n278 = Concatenate Strings("<" ("string"), w705, w706, w708, "</" ("string"), w705, w706) -> (w709:string)
                    }
                  }
                }
                frame "U32" {
                  n279 = Get Variant Attribute(Variant=w717, name=w712) -> (duplicate Variant=w718:variant)  [unwired: 2 in, 3 out]
                  n280 = Equal?(x=w714, y="") -> (x = y?=w716:bool)
                  n281 = Variant To Data(Variant=w718, type=u32 0) -> (data=w720:cluster{})  [unwired: 1 in, 1 out]
                  n282 = Number To Decimal String(number=w720) -> (decimal integer string=w713:string)  [unwired: 1 in]
                  n283 = case shown="True" w716 {
                    tunnel: w712 -> [w724 w729]
                    tunnel: w714 -> [w721 _]
                    tunnel: w713 -> [w723 w732]
                    tunnel: [w722 w733] -> w711
                    frame False {
                      w727 = ">" ("string")
                      n284 = call <vilib>:"Space Constant.vi"() -> ("String"=w728:string)
                      n285 = Concatenate Strings("<" ("string"), w724, w728, w721, w727, w723, "</" ("string"), w724, w727) -> (w722:string)
                    }
                    frame True {
                      w730 = ">" ("string")
                      n286 = Concatenate Strings("<" ("string"), w729, w730, w732, "</" ("string"), w729, w730) -> (w733:string)
                    }
                  }
                }
                frame "U64" {
                  n287 = Get Variant Attribute(Variant=w741, name=w736) -> (duplicate Variant=w742:variant)  [unwired: 2 in, 3 out]
                  n288 = Equal?(x=w738, y="") -> (x = y?=w740:bool)
                  n289 = Variant To Data(Variant=w742, type=u64 0) -> (data=w744:cluster{})  [unwired: 1 in, 1 out]
                  n290 = Number To Decimal String(number=w744) -> (decimal integer string=w737:string)  [unwired: 1 in]
                  n291 = case shown="True" w740 {
                    tunnel: w736 -> [w748 w753]
                    tunnel: w738 -> [w745 _]
                    tunnel: w737 -> [w747 w756]
                    tunnel: [w746 w757] -> w735
                    frame False {
                      w751 = ">" ("string")
                      n292 = call <vilib>:"Space Constant.vi"() -> ("String"=w752:string)
                      n293 = Concatenate Strings("<" ("string"), w748, w752, w745, w751, w747, "</" ("string"), w748, w751) -> (w746:string)
                    }
                    frame True {
                      w754 = ">" ("string")
                      n294 = Concatenate Strings("<" ("string"), w753, w754, w756, "</" ("string"), w753, w754) -> (w757:string)
                    }
                  }
                }
                frame "Single Float" {
                  n295 = Get Variant Attribute(Variant=w767, name=w760) -> (duplicate Variant=w768:variant)  [unwired: 2 in, 3 out]
                  n296 = Equal?(x=w762, y="") -> (x = y?=w764:bool)
                  n297 = Variant To Data(Variant=w768, type=sgl 0.0) -> (data=w765:cluster{})  [unwired: 1 in, 1 out]
                  n298 = Format Into String(format string="%#f", w765) -> (resulting string=w761:string)  [unwired: 2 in, 1 out]
                  n299 = case shown="True" w764 {
                    tunnel: w760 -> [w773 w778]
                    tunnel: w762 -> [w770 _]
                    tunnel: w761 -> [w772 w781]
                    tunnel: [w771 w782] -> w759
                    frame False {
                      w776 = ">" ("string")
                      n300 = call <vilib>:"Space Constant.vi"() -> ("String"=w777:string)
                      n301 = Concatenate Strings("<" ("string"), w773, w777, w770, w776, w772, "</" ("string"), w773, w776) -> (w771:string)
                    }
                    frame True {
                      w779 = ">" ("string")
                      n302 = Concatenate Strings("<" ("string"), w778, w779, w781, "</" ("string"), w778, w779) -> (w782:string)
                    }
                  }
                }
                frame "Double Float" {
                  n303 = Get Variant Attribute(Variant=w792, name=w785) -> (duplicate Variant=w793:variant)  [unwired: 2 in, 3 out]
                  n304 = Equal?(x=w787, y="") -> (x = y?=w789:bool)
                  n305 = Variant To Data(Variant=w793, type=0.0) -> (data=w790:cluster{})  [unwired: 1 in, 1 out]
                  n306 = Format Into String(format string="%#f", w790) -> (resulting string=w786:string)  [unwired: 2 in, 1 out]
                  n307 = case shown="True" w789 {
                    tunnel: w785 -> [w798 w803]
                    tunnel: w787 -> [w795 _]
                    tunnel: w786 -> [w797 w806]
                    tunnel: [w796 w807] -> w784
                    frame False {
                      w801 = ">" ("string")
                      n308 = call <vilib>:"Space Constant.vi"() -> ("String"=w802:string)
                      n309 = Concatenate Strings("<" ("string"), w798, w802, w795, w801, w797, "</" ("string"), w798, w801) -> (w796:string)
                    }
                    frame True {
                      w804 = ">" ("string")
                      n310 = Concatenate Strings("<" ("string"), w803, w804, w806, "</" ("string"), w803, w804) -> (w807:string)
                    }
                  }
                }
                frame "Extended Float" {
                  n311 = Get Variant Attribute(Variant=w817, name=w810) -> (duplicate Variant=w818:variant)  [unwired: 2 in, 3 out]
                  n312 = Equal?(x=w812, y="") -> (x = y?=w814:bool)
                  n313 = Variant To Data(Variant=w818, type=ext 0.0) -> (data=w815:cluster{})  [unwired: 1 in, 1 out]
                  n314 = Format Into String(format string="%#f", w815) -> (resulting string=w811:string)  [unwired: 2 in, 1 out]
                  n315 = case shown="True" w814 {
                    tunnel: w810 -> [w823 w828]
                    tunnel: w812 -> [w820 _]
                    tunnel: w811 -> [w822 w831]
                    tunnel: [w821 w832] -> w809
                    frame False {
                      w826 = ">" ("string")
                      n316 = call <vilib>:"Space Constant.vi"() -> ("String"=w827:string)
                      n317 = Concatenate Strings("<" ("string"), w823, w827, w820, w826, w822, "</" ("string"), w823, w826) -> (w821:string)
                    }
                    frame True {
                      w829 = ">" ("string")
                      n318 = Concatenate Strings("<" ("string"), w828, w829, w831, "</" ("string"), w828, w829) -> (w832:string)
                    }
                  }
                }
                frame "Single Complex" {
                  n319 = Get Variant Attribute(Variant=w840, name=w835) -> (duplicate Variant=w841:variant)  [unwired: 2 in, 3 out]
                  n320 = Equal?(x=w837, y="") -> (x = y?=w839:bool)
                  n321 = Variant To Data(Variant=w841, type=csg 0.0+0.0i ("number 3")) -> (data=w843:cluster{})  [unwired: 1 in, 1 out]
                  n322 = Format Value(value (0)=w843) -> (output string=w836:string)  [unwired: 2 in]
                  n323 = case shown="True" w839 {
                    tunnel: w835 -> [w847 w852]
                    tunnel: w837 -> [w844 _]
                    tunnel: w836 -> [w846 w855]
                    tunnel: [w845 w856] -> w834
                    frame False {
                      w850 = ">" ("string")
                      n324 = call <vilib>:"Space Constant.vi"() -> ("String"=w851:string)
                      n325 = Concatenate Strings("<" ("string"), w847, w851, w844, w850, w846, "</" ("string"), w847, w850) -> (w845:string)
                    }
                    frame True {
                      w853 = ">" ("string")
                      n326 = Concatenate Strings("<" ("string"), w852, w853, w855, "</" ("string"), w852, w853) -> (w856:string)
                    }
                  }
                }
                frame "Double Complex" {
                  n327 = Get Variant Attribute(Variant=w864, name=w859) -> (duplicate Variant=w865:variant)  [unwired: 2 in, 3 out]
                  n328 = Equal?(x=w861, y="") -> (x = y?=w863:bool)
                  n329 = Variant To Data(Variant=w865, type=cdb 0.0+0.0i ("number 3")) -> (data=w867:cluster{})  [unwired: 1 in, 1 out]
                  n330 = Format Value(value (0)=w867) -> (output string=w860:string)  [unwired: 2 in]
                  n331 = case shown="True" w863 {
                    tunnel: w859 -> [w871 w876]
                    tunnel: w861 -> [w868 _]
                    tunnel: w860 -> [w870 w879]
                    tunnel: [w869 w880] -> w858
                    frame False {
                      w874 = ">" ("string")
                      n332 = call <vilib>:"Space Constant.vi"() -> ("String"=w875:string)
                      n333 = Concatenate Strings("<" ("string"), w871, w875, w868, w874, w870, "</" ("string"), w871, w874) -> (w869:string)
                    }
                    frame True {
                      w877 = ">" ("string")
                      n334 = Concatenate Strings("<" ("string"), w876, w877, w879, "</" ("string"), w876, w877) -> (w880:string)
                    }
                  }
                }
                frame "Extended Complex" {
                  n335 = Get Variant Attribute(Variant=w888, name=w883) -> (duplicate Variant=w889:variant)  [unwired: 2 in, 3 out]
                  n336 = Equal?(x=w885, y="") -> (x = y?=w887:bool)
                  n337 = Variant To Data(Variant=w889, type=cxt 0.0+0.0i ("number 3")) -> (data=w890:cluster{})  [unwired: 1 in, 1 out]
                  n338 = Format Value(value (0)=w890) -> (output string=w884:string)  [unwired: 2 in]
                  n339 = case shown="True" w887 {
                    tunnel: w883 -> [w895 w900]
                    tunnel: w885 -> [w892 _]
                    tunnel: w884 -> [w894 w903]
                    tunnel: [w893 w904] -> w882
                    frame False {
                      w898 = ">" ("string")
                      n340 = call <vilib>:"Space Constant.vi"() -> ("String"=w899:string)
                      n341 = Concatenate Strings("<" ("string"), w895, w899, w892, w898, w894, "</" ("string"), w895, w898) -> (w893:string)
                    }
                    frame True {
                      w901 = ">" ("string")
                      n342 = Concatenate Strings("<" ("string"), w900, w901, w903, "</" ("string"), w900, w901) -> (w904:string)
                    }
                  }
                }
                frame "Boolean" {
                  n343 = Get Variant Attribute(Variant=w912, name=w907) -> (duplicate Variant=w913:variant)  [unwired: 2 in, 3 out]
                  n344 = Equal?(x=w909, y="") -> (x = y?=w911:bool)
                  n345 = Variant To Data(Variant=w913, type=TRUE) -> (data=w916:cluster{})  [unwired: 1 in, 1 out]
                  n346 = Boolean To (0,1)(Boolean=w916) -> (0, 1=w914:i16)
                  n347 = Number To Decimal String(number=w914) -> (decimal integer string=w908:string)  [unwired: 1 in]
                  n348 = case shown="True" w911 {
                    tunnel: w907 -> [w920 w925]
                    tunnel: w909 -> [w917 _]
                    tunnel: w908 -> [w919 w928]
                    tunnel: [w918 w929] -> w906
                    frame False {
                      w923 = ">" ("string")
                      n349 = call <vilib>:"Space Constant.vi"() -> ("String"=w924:string)
                      n350 = Concatenate Strings("<" ("string"), w920, w924, w917, w923, w919, "</" ("string"), w920, w923) -> (w918:string)
                    }
                    frame True {
                      w926 = ">" ("string")
                      n351 = Concatenate Strings("<" ("string"), w925, w926, w928, "</" ("string"), w925, w926) -> (w929:string)
                    }
                  }
                }
                frame "Array" {
                  n352 = call <vilib>:"GetArrayInfo.vi"("Variant"=w937) -> ("ArrayElement"=w939:variant)  [unwired: 7 in, 3 out]
                  n353 = Equal?(x=w932, y="") -> (x = y?=w935:bool)
                  n354 = call <vilib>:"GetTypeInfo.vi"("Variant"=w939) -> ("Type Enum"=w938:T6)  [unwired: 6 in, 4 out]
                  n355 = case shown="\"Double Float\"" w938 {
                    tunnel: w937 -> [w960 w975 w988 w1004 w1019 w1036 w1051 w1068 w1083 w1100 w1118 w1135 w1151 w1167 w1185]
                    tunnel: [w955 w973 w986 w1002 w1020 w1034 w1052 w1066 w1085 w1101 w1116 w1133 w1149 w1165 w1181] -> w933
                    tunnel: w932 -> [w954 w970 w987 w1003 w1018 w1035 w1050 w1067 w1082 w1099 w1117 w1134 w1150 w1166 w1184]
                    frame "I8" {
                      n356 = Get Variant Attribute(Variant=w960, name=w954) -> (duplicate Variant=w959:variant)  [unwired: 2 in, 3 out]
                      n357 = Variant To Data(Variant=w959, type=u8[] [] ("Array")) -> (data=w957:cluster{})  [unwired: 1 in, 1 out]
                      n358 = while {
                        tunnel: w957 -> [w969] mode=indexing
                        tunnel: w957 -> [w968]
                        shift-right: [w961] -> w955
                        shift-left: "" -> [w962]
                        i -> [w966]
                        stop <- w965 stop-if-true
                        n359 = Array Size(array=w968) -> (size(s)=w967:i32)
                        n360 = Number To Decimal String(number=w969) -> (decimal integer string=w964:string)  [unwired: 1 in]
                        n361 = call <vilib>:"Space Constant.vi"() -> ("String"=w963:string)
                        n362 = Equal?(x=w967, y=w966) -> (x = y?=w965:bool)
                        n363 = Concatenate Strings(w962, w964, w963) -> (w961:string)
                      }
                    }
                    frame "I16" {
                      n364 = Get Variant Attribute(Variant=w975, name=w970) -> (duplicate Variant=w972:variant)  [unwired: 2 in, 3 out]
                      n365 = Variant To Data(Variant=w972, type=i16[] [] ("Array")) -> (data=w971:cluster{})  [unwired: 1 in, 1 out]
                      n366 = while {
                        tunnel: w971 -> [w985] mode=indexing
                        shift-right: [w978] -> w973
                        shift-left: "" -> [w979]
                        tunnel: w971 -> [w977]
                        i -> [w983]
                        stop <- w982 stop-if-true
                        n367 = Array Size(array=w977) -> (size(s)=w984:i32)
                        n368 = Number To Decimal String(number=w985) -> (decimal integer string=w981:string)  [unwired: 1 in]
                        n369 = call <vilib>:"Space Constant.vi"() -> ("String"=w980:string)
                        n370 = Equal?(x=w984, y=w983) -> (x = y?=w982:bool)
                        n371 = Concatenate Strings(w979, w981, w980) -> (w978:string)
                      }
                    }
                    frame "I32" {
                      n372 = Get Variant Attribute(Variant=w988, name=w987) -> (duplicate Variant=w990:variant)  [unwired: 2 in, 3 out]
                      n373 = Variant To Data(Variant=w990, type=i16[] [] ("Array")) -> (data=w989:cluster{})  [unwired: 1 in, 1 out]
                      n374 = while {
                        tunnel: w989 -> [w1001] mode=indexing
                        shift-right: [w994] -> w986
                        shift-left: "" -> [w995]
                        tunnel: w989 -> [w993]
                        i -> [w999]
                        stop <- w998 stop-if-true
                        n375 = Array Size(array=w993) -> (size(s)=w1000:i32)
                        n376 = Number To Decimal String(number=w1001) -> (decimal integer string=w997:string)  [unwired: 1 in]
                        n377 = call <vilib>:"Space Constant.vi"() -> ("String"=w996:string)
                        n378 = Equal?(x=w1000, y=w999) -> (x = y?=w998:bool)
                        n379 = Concatenate Strings(w995, w997, w996) -> (w994:string)
                      }
                    }
                    frame "I64" {
                      n380 = Get Variant Attribute(Variant=w1004, name=w1003) -> (duplicate Variant=w1006:variant)  [unwired: 2 in, 3 out]
                      n381 = Variant To Data(Variant=w1006, type=i64[] [] ("Array")) -> (data=w1005:cluster{})  [unwired: 1 in, 1 out]
                      n382 = while {
                        tunnel: w1005 -> [w1017] mode=indexing
                        shift-right: [w1010] -> w1002
                        shift-left: "" -> [w1011]
                        tunnel: w1005 -> [w1009]
                        i -> [w1015]
                        stop <- w1014 stop-if-true
                        n383 = Array Size(array=w1009) -> (size(s)=w1016:i32)
                        n384 = Number To Decimal String(number=w1017) -> (decimal integer string=w1013:string)  [unwired: 1 in]
                        n385 = call <vilib>:"Space Constant.vi"() -> ("String"=w1012:string)
                        n386 = Equal?(x=w1016, y=w1015) -> (x = y?=w1014:bool)
                        n387 = Concatenate Strings(w1011, w1013, w1012) -> (w1010:string)
                      }
                    }
                    frame "U8" {
                      n388 = Get Variant Attribute(Variant=w1019, name=w1018) -> (duplicate Variant=w1022:variant)  [unwired: 2 in, 3 out]
                      n389 = Variant To Data(Variant=w1022, type=u8[] [] ("Array")) -> (data=w1021:cluster{})  [unwired: 1 in, 1 out]
                      n390 = while {
                        tunnel: w1021 -> [w1033] mode=indexing
                        shift-right: [w1026] -> w1020
                        shift-left: "" -> [w1027]
                        tunnel: w1021 -> [w1025]
                        i -> [w1031]
                        stop <- w1030 stop-if-true
                        n391 = Array Size(array=w1025) -> (size(s)=w1032:i32)
                        n392 = Number To Decimal String(number=w1033) -> (decimal integer string=w1029:string)  [unwired: 1 in]
                        n393 = call <vilib>:"Space Constant.vi"() -> ("String"=w1028:string)
                        n394 = Equal?(x=w1032, y=w1031) -> (x = y?=w1030:bool)
                        n395 = Concatenate Strings(w1027, w1029, w1028) -> (w1026:string)
                      }
                    }
                    frame "U16" {
                      n396 = Get Variant Attribute(Variant=w1036, name=w1035) -> (duplicate Variant=w1038:variant)  [unwired: 2 in, 3 out]
                      n397 = Variant To Data(Variant=w1038, type=u16[] [] ("Array")) -> (data=w1037:cluster{})  [unwired: 1 in, 1 out]
                      n398 = while {
                        tunnel: w1037 -> [w1049] mode=indexing
                        shift-right: [w1042] -> w1034
                        shift-left: "" -> [w1043]
                        tunnel: w1037 -> [w1041]
                        i -> [w1047]
                        stop <- w1046 stop-if-true
                        n399 = Array Size(array=w1041) -> (size(s)=w1048:i32)
                        n400 = Number To Decimal String(number=w1049) -> (decimal integer string=w1045:string)  [unwired: 1 in]
                        n401 = call <vilib>:"Space Constant.vi"() -> ("String"=w1044:string)
                        n402 = Equal?(x=w1048, y=w1047) -> (x = y?=w1046:bool)
                        n403 = Concatenate Strings(w1043, w1045, w1044) -> (w1042:string)
                      }
                    }
                    frame "U32" {
                      n404 = Get Variant Attribute(Variant=w1051, name=w1050) -> (duplicate Variant=w1054:variant)  [unwired: 2 in, 3 out]
                      n405 = Variant To Data(Variant=w1054, type=u32[] [] ("Array")) -> (data=w1053:cluster{})  [unwired: 1 in, 1 out]
                      n406 = while {
                        tunnel: w1053 -> [w1065] mode=indexing
                        shift-right: [w1058] -> w1052
                        shift-left: "" -> [w1059]
                        tunnel: w1053 -> [w1057]
                        i -> [w1063]
                        stop <- w1062 stop-if-true
                        n407 = Array Size(array=w1057) -> (size(s)=w1064:i32)
                        n408 = Number To Decimal String(number=w1065) -> (decimal integer string=w1061:string)  [unwired: 1 in]
                        n409 = call <vilib>:"Space Constant.vi"() -> ("String"=w1060:string)
                        n410 = Equal?(x=w1064, y=w1063) -> (x = y?=w1062:bool)
                        n411 = Concatenate Strings(w1059, w1061, w1060) -> (w1058:string)
                      }
                    }
                    frame "U64" {
                      n412 = Get Variant Attribute(Variant=w1068, name=w1067) -> (duplicate Variant=w1070:variant)  [unwired: 2 in, 3 out]
                      n413 = Variant To Data(Variant=w1070, type=u64[] [] ("Array")) -> (data=w1069:cluster{})  [unwired: 1 in, 1 out]
                      n414 = while {
                        tunnel: w1069 -> [w1081] mode=indexing
                        shift-right: [w1074] -> w1066
                        shift-left: "" -> [w1075]
                        tunnel: w1069 -> [w1073]
                        i -> [w1079]
                        stop <- w1078 stop-if-true
                        n415 = Array Size(array=w1073) -> (size(s)=w1080:i32)
                        n416 = Number To Decimal String(number=w1081) -> (decimal integer string=w1077:string)  [unwired: 1 in]
                        n417 = call <vilib>:"Space Constant.vi"() -> ("String"=w1076:string)
                        n418 = Equal?(x=w1080, y=w1079) -> (x = y?=w1078:bool)
                        n419 = Concatenate Strings(w1075, w1077, w1076) -> (w1074:string)
                      }
                    }
                    frame "Single Float" {
                      n420 = Get Variant Attribute(Variant=w1083, name=w1082) -> (duplicate Variant=w1086:variant)  [unwired: 2 in, 3 out]
                      n421 = Variant To Data(Variant=w1086, type=sgl[] [] ("Array")) -> (data=w1084:cluster{})  [unwired: 1 in, 1 out]
                      n422 = while {
                        tunnel: w1084 -> [w1090] mode=indexing
                        shift-right: [w1093] -> w1085
                        shift-left: "" -> [w1094]
                        tunnel: w1084 -> [w1092]
                        i -> [w1097]
                        stop <- w1096 stop-if-true
                        n423 = Array Size(array=w1092) -> (size(s)=w1098:i32)
                        n424 = Format Into String(format string="%#f", w1090) -> (resulting string=w1089:string)  [unwired: 2 in, 1 out]
                        n425 = Equal?(x=w1098, y=w1097) -> (x = y?=w1096:bool)
                        n426 = call <vilib>:"Space Constant.vi"() -> ("String"=w1095:string)
                        n427 = Concatenate Strings(w1094, w1089, w1095) -> (w1093:string)
                      }
                    }
                    frame "Double Float" {
                      n428 = Get Variant Attribute(Variant=w1100, name=w1099) -> (duplicate Variant=w1103:variant)  [unwired: 2 in, 3 out]
                      n429 = Variant To Data(Variant=w1103, type=dbl[] [] ("Array")) -> (data=w1102:cluster{})  [unwired: 1 in, 1 out]
                      n430 = while {
                        tunnel: w1102 -> [w1107] mode=indexing
                        shift-right: [w1110] -> w1101
                        shift-left: "" -> [w1111]
                        tunnel: w1102 -> [w1109]
                        i -> [w1114]
                        stop <- w1113 stop-if-true
                        n431 = Array Size(array=w1109) -> (size(s)=w1115:i32)
                        n432 = Format Into String(format string="%f", w1107) -> (resulting string=w1106:string)  [unwired: 2 in, 1 out]
                        n433 = Equal?(x=w1115, y=w1114) -> (x = y?=w1113:bool)
                        n434 = call <vilib>:"Space Constant.vi"() -> ("String"=w1112:string)
                        n435 = Concatenate Strings(w1111, w1106, w1112) -> (w1110:string)
                      }
                    }
                    frame "Extended Float" {
                      n436 = Get Variant Attribute(Variant=w1118, name=w1117) -> (duplicate Variant=w1120:variant)  [unwired: 2 in, 3 out]
                      n437 = Variant To Data(Variant=w1120, type=ext[] [] ("Array")) -> (data=w1119:cluster{})  [unwired: 1 in, 1 out]
                      n438 = while {
                        tunnel: w1119 -> [w1124] mode=indexing
                        shift-right: [w1127] -> w1116
                        shift-left: "" -> [w1128]
                        tunnel: w1119 -> [w1126]
                        i -> [w1131]
                        stop <- w1130 stop-if-true
                        n439 = Array Size(array=w1126) -> (size(s)=w1132:i32)
                        n440 = Format Into String(format string="%#f", w1124) -> (resulting string=w1123:string)  [unwired: 2 in, 1 out]
                        n441 = Equal?(x=w1132, y=w1131) -> (x = y?=w1130:bool)
                        n442 = call <vilib>:"Space Constant.vi"() -> ("String"=w1129:string)
                        n443 = Concatenate Strings(w1128, w1123, w1129) -> (w1127:string)
                      }
                    }
                    frame "Single Complex" {
                      n444 = Get Variant Attribute(Variant=w1135, name=w1134) -> (duplicate Variant=w1137:variant)  [unwired: 2 in, 3 out]
                      n445 = Variant To Data(Variant=w1137, type=csg[] [] ("Array")) -> (data=w1136:cluster{})  [unwired: 1 in, 1 out]
                      n446 = while {
                        tunnel: w1136 -> [w1141] mode=indexing
                        shift-right: [w1143] -> w1133
                        shift-left: "" -> [w1144]
                        tunnel: w1136 -> [w1142]
                        i -> [w1147]
                        stop <- w1146 stop-if-true
                        n447 = Array Size(array=w1142) -> (size(s)=w1148:i32)
                        n448 = Format Value(value (0)=w1141) -> (output string=w1140:string)  [unwired: 2 in]
                        n449 = call <vilib>:"Space Constant.vi"() -> ("String"=w1145:string)
                        n450 = Equal?(x=w1148, y=w1147) -> (x = y?=w1146:bool)
                        n451 = Concatenate Strings(w1144, w1140, w1145) -> (w1143:string)
                      }
                    }
                    frame "Double Complex" {
                      n452 = Get Variant Attribute(Variant=w1151, name=w1150) -> (duplicate Variant=w1153:variant)  [unwired: 2 in, 3 out]
                      n453 = Variant To Data(Variant=w1153, type=cdb[] [] ("Array")) -> (data=w1152:cluster{})  [unwired: 1 in, 1 out]
                      n454 = while {
                        tunnel: w1152 -> [w1157] mode=indexing
                        shift-right: [w1159] -> w1149
                        shift-left: "" -> [w1160]
                        tunnel: w1152 -> [w1158]
                        i -> [w1163]
                        stop <- w1162 stop-if-true
                        n455 = Array Size(array=w1158) -> (size(s)=w1164:i32)
                        n456 = Format Value(value (0)=w1157) -> (output string=w1156:string)  [unwired: 2 in]
                        n457 = call <vilib>:"Space Constant.vi"() -> ("String"=w1161:string)
                        n458 = Equal?(x=w1164, y=w1163) -> (x = y?=w1162:bool)
                        n459 = Concatenate Strings(w1160, w1156, w1161) -> (w1159:string)
                      }
                    }
                    frame "Extended Complex" {
                      n460 = Get Variant Attribute(Variant=w1167, name=w1166) -> (duplicate Variant=w1169:variant)  [unwired: 2 in, 3 out]
                      n461 = Variant To Data(Variant=w1169, type=cxt[] [] ("Array")) -> (data=w1168:cluster{})  [unwired: 1 in, 1 out]
                      n462 = while {
                        tunnel: w1168 -> [w1173] mode=indexing
                        shift-right: [w1175] -> w1165
                        shift-left: "" -> [w1176]
                        tunnel: w1168 -> [w1174]
                        i -> [w1179]
                        stop <- w1178 stop-if-true
                        n463 = Array Size(array=w1174) -> (size(s)=w1180:i32)
                        n464 = Format Value(value (0)=w1173) -> (output string=w1172:string)  [unwired: 2 in]
                        n465 = call <vilib>:"Space Constant.vi"() -> ("String"=w1177:string)
                        n466 = Equal?(x=w1180, y=w1179) -> (x = y?=w1178:bool)
                        n467 = Concatenate Strings(w1176, w1172, w1177) -> (w1175:string)
                      }
                    }
                    frame "String", Default {
                      n468 = Get Variant Attribute(Variant=w1185, name=w1184) -> (duplicate Variant=w1186:variant)  [unwired: 2 in, 3 out]
                      n469 = Variant To Data(Variant=w1186, type=string[] [] ("Array")) -> (data=w1182:cluster{})  [unwired: 1 in, 1 out]
                      n470 = while {
                        tunnel: w1182 -> [w1188] mode=indexing
                        shift-right: [w1190] -> w1181
                        shift-left: "" -> [w1191]
                        tunnel: w1182 -> [w1189]
                        i -> [w1194]
                        stop <- w1193 stop-if-true
                        n471 = call <vilib>:"Space Constant.vi"() -> ("String"=w1192:string)
                        n472 = Array Size(array=w1189) -> (size(s)=w1195:i32)
                        n473 = Concatenate Strings(w1191, w1188, w1192) -> (w1190:string)
                        n474 = Equal?(x=w1195, y=w1194) -> (x = y?=w1193:bool)
                      }
                    }
                  }
                  n475 = case shown="True" w935 {
                    tunnel: w932 -> [w943 w948]
                    tunnel: w931 -> [w940 _]
                    tunnel: w933 -> [w942 w951]
                    tunnel: [w941 w952] -> w936
                    frame False {
                      w946 = ">" ("string")
                      n476 = call <vilib>:"Space Constant.vi"() -> ("String"=w947:string)
                      n477 = Concatenate Strings("<" ("string"), w943, w947, w940, w946, w942, "</" ("string"), w943, w946) -> (w941:string)
                    }
                    frame True {
                      w949 = ">" ("string")
                      n478 = Concatenate Strings("<" ("string"), w948, w949, w951, "</" ("string"), w948, w949) -> (w952:string)
                    }
                  }
                }
                frame "String", Default {
                  n479 = Get Variant Attribute(Variant=w1202, name=w1200) -> (duplicate Variant=w1203:variant)  [unwired: 2 in, 3 out]
                  n480 = Equal?(x=w1198, y="") -> (x = y?=w1199:bool)
                  n481 = Variant To Data(Variant=w1203, type="") -> (data=w1201:cluster{})  [unwired: 1 in, 1 out]
                  n482 = case shown="True" w1199 {
                    tunnel: w1200 -> [w1208 w1213]
                    tunnel: w1198 -> [w1205 _]
                    tunnel: w1201 -> [w1207 w1216]
                    tunnel: [w1206 w1217] -> w1196
                    frame False {
                      w1211 = ">" ("string")
                      n483 = call <vilib>:"Space Constant.vi"() -> ("String"=w1212:string)
                      n484 = Concatenate Strings("<" ("string"), w1208, w1212, w1205, w1211, w1207, "</" ("string"), w1208, w1211) -> (w1206:string)
                    }
                    frame True {
                      w1214 = ">" ("string")
                      n485 = Concatenate Strings("<" ("string"), w1213, w1214, w1216, "</" ("string"), w1213, w1214) -> (w1217:string)
                    }
                  }
                }
                frame "Fixed Point" {
                  n486 = Get Variant Attribute(Variant=w1228, name=w1220) -> (duplicate Variant=w1229:variant)  [unwired: 2 in, 3 out]
                  n487 = Equal?(x=w1222, y="") -> (x = y?=w1224:bool)
                  n488 = Variant To Data(Variant=w1229, type=fxp<+,1,1> 0.0) -> (data=w1226:cluster{})  [unwired: 1 in, 1 out]
                  n489 = Format Into String(format string="%#f", w1226) -> (resulting string=w1221:string)  [unwired: 2 in, 1 out]
                  n490 = case shown="True" w1224 {
                    tunnel: w1220 -> [w1233 w1238]
                    tunnel: w1222 -> [w1230 _]
                    tunnel: w1221 -> [w1232 w1241]
                    tunnel: [w1231 w1242] -> w1219
                    frame False {
                      w1236 = ">" ("string")
                      n491 = call <vilib>:"Space Constant.vi"() -> ("String"=w1237:string)
                      n492 = Concatenate Strings("<" ("string"), w1233, w1237, w1230, w1236, w1232, "</" ("string"), w1233, w1236) -> (w1231:string)
                    }
                    frame True {
                      w1239 = ">" ("string")
                      n493 = Concatenate Strings("<" ("string"), w1238, w1239, w1241, "</" ("string"), w1238, w1239) -> (w1242:string)
                    }
                  }
                }
              }
            }
            n494 = Concatenate Strings(w555, w557, w554) -> (w558:string)
            n495 = local write "XML-String-out"(w558) -> ()
          }
          frame "Set" {
            n496 = local read "Database"() -> (w1257:string)
            n497 = local read "error in (no error)"() -> (w1254:errorcluster)
            n498 = local read "XML-String-out"() -> (w1250:string)
            n499 = Wait (ms)(milliseconds to wait=u32 1000) -> ()  [unwired: 1 out]
            n500 = call-poly <vilib>:"DB Tools Open Connection.vi"("error in (no error)"=w1254, "connection information"=w1257) -> ("error out"=w1247:errorcluster, "connection reference"=w1248:T4)  [unwired: 6 in]
            n501 = Unbundle By Name(w1247) -> ("status"=w1253:bool, "code"=w1246:i32, "source"=w1251:string)
            n502 = local read "exp_id"() -> (w1249:i32)
            n503 = case shown="True" w1253 {
              selector: w1253 -> [w1298 _]
              tunnel: w1246 -> [w1297 _]
              tunnel: w1251 -> [w1275 w1321]
              tunnel: [w1296 errorcluster {"status"=FALSE, "code"=0, "source"=""} ("error in (no error)")] -> w1244
              tunnel: w1248 -> [w1295 w1334]
              tunnel: [w1293 w1325] -> w1245
              tunnel: w1250 -> [w1285 w1333]
              tunnel: w1249 -> [w1284 w1332]
              frame False {
                w1259 = "' WHERE exp_id =" ("string")
                w1277 = "\t"
                w1260 = " WHERE exp_id ="
                n504 = Get Date/Time In Seconds() -> (seconds since 1Jan1904=w1267:timestamp)
                n505 = local read "submit_time"() -> (w1264:timestamp)
                n506 = local read "exec_time"() -> (w1265:timestamp)
                n507 = Subtract(x=w1267, y=w1265) -> (x-y=w1273:dbl)
                n508 = Subtract(x=w1267, y=w1264) -> (x-y=w1272:dbl)
                n509 = Number To Decimal String(number=w1284) -> (decimal integer string=w1268:string)  [unwired: 1 in]
                n510 = Format Date/Time String(seconds (now)=w1267) -> (date/time string=w1278:string)  [unwired: 2 in]
                n511 = local read "Status"() -> (w1282:string)
                n512 = To Long Integer(number=w1273) -> (32bit integer=w1262:i32)
                n513 = To Long Integer(number=w1272) -> (32bit integer=w1261:i32)
                n514 = Format Date/Time String(seconds (now)=w1267) -> (date/time string=w1288:string)  [unwired: 2 in]
                n515 = Number To Decimal String(number=w1262) -> (decimal integer string=w1266:string)  [unwired: 1 in]
                n516 = Number To Decimal String(number=w1261) -> (decimal integer string=w1270:string)  [unwired: 1 in]
                n517 = Concatenate Strings(w1282, "Job completed!! exp_id = " ("string"), w1268, w1277, w1277, w1278, "\r\n") -> (w1281:string)
                n518 = Concatenate Strings("UPDATE dbo.JobRecord SET end_time = '", w1288, w1259, w1268) -> (w1292:string)
                n519 = Concatenate Strings("UPDATE dbo.JobRecord SET error_report = '" ("string"), w1275, w1259, w1268) -> (w1274:string)
                n520 = Concatenate Strings("UPDATE dbo.JobRecord SET exec_elapsed = ", w1266, w1260, w1268) -> (w1263:string)
                n521 = Concatenate Strings("UPDATE dbo.JobRecord SET job_elapsed = ", w1270, w1260, w1268) -> (w1258:string)
                n522 = local write "Status"(w1281) -> ()
                n523 = Concatenate Strings("UPDATE dbo.JobRecord SET experiment_results = '", w1285, w1259, w1268) -> (w1290:string)
                n524 = Concatenate Strings("UPDATE dbo.JobRecord SET job_status = 'COMPLETE' WHERE exp_id =", w1268) -> (w1291:string)
                n525 = Concatenate Strings(w1290, w1291, w1292, w1274, w1263, w1258) -> (w1283:string)
                n526 = call-poly <vilib>:"DB Tools Execute Query.vi"("SQL query"=w1283, "connection reference"=w1295) -> ("recordset reference"=w1294:T5)  [unwired: 6 in, 1 out]
                n527 = call-poly <vilib>:"DB Tools Free Object.vi"("recordset reference"=w1294) -> ("connection reference"=w1293:T4)  [unwired: 9 in, 1 out]
                n528 = Bundle(w1298, "code"=w1297, "source"=w1275) -> (w1296:cluster{bool, "code":i32, "source":string})  [unwired: 1 in]
              }
              frame True {
                w1300 = "WHERE exp_id =" ("string")
                w1319 = "\t"
                w1304 = "' WHERE exp_id ="
                n529 = Get Date/Time In Seconds() -> (seconds since 1Jan1904=w1309:timestamp)
                n530 = local read "submit_time"() -> (w1308:timestamp)
                n531 = local read "exec_time"() -> (w1318:timestamp)
                n532 = Format Date/Time String(seconds (now)=w1309) -> (date/time string=w1316:string)  [unwired: 2 in]
                n533 = Number To Decimal String(number=w1332) -> (decimal integer string=w1303:string)  [unwired: 1 in]
                n534 = Subtract(x=w1309, y=w1318) -> (x-y=w1313:dbl)
                n535 = Subtract(x=w1309, y=w1308) -> (x-y=w1307:dbl)
                n536 = local read "Status"() -> (w1323:string)
                n537 = call <vilib>:"Space Constant.vi"() -> ("String"=w1314:string)
                n538 = To Long Integer(number=w1313) -> (32bit integer=w1301:i32)
                n539 = To Long Integer(number=w1307) -> (32bit integer=w1302:i32)
                n540 = Concatenate Strings(w1323, "Error occurred: " ("Status"), w1321, "exp_id = " ("string"), w1303, w1319, w1319, w1314, w1316, "\r\n") -> (w1322:string)
                n541 = Number To Decimal String(number=w1302) -> (decimal integer string=w1305:string)  [unwired: 1 in]
                n542 = local write "Status"(w1322) -> ()
                n543 = Format Date/Time String(seconds (now)=w1309) -> (date/time string=w1315:string)  [unwired: 2 in]
                n544 = Number To Decimal String(number=w1301) -> (decimal integer string=w1311:string)  [unwired: 1 in]
                n545 = Concatenate Strings("UPDATE dbo.JobRecord SET error_report = '" ("string"), w1321, w1304, w1303) -> (w1327:string)
                n546 = Concatenate Strings("UPDATE dbo.JobRecord SET end_time = '", w1314, w1315, w1304, w1303) -> (w1329:string)
                n547 = Concatenate Strings("UPDATE dbo.JobRecord SET exec_elapsed = ", w1311, w1300, w1303) -> (w1310:string)
                n548 = Concatenate Strings("UPDATE dbo.JobRecord SET job_elapsed = ", w1305, w1300, w1303) -> (w1299:string)
                n549 = Concatenate Strings("UPDATE dbo.JobRecord SET experiment_results = '", w1333, w1304, w1303) -> (w1339:string)
                n550 = Concatenate Strings("UPDATE dbo.JobRecord SET job_status = 'IN PROGRESS' WHERE exp_id =", w1303) -> (w1340:string)
                n551 = Concatenate Strings("UPDATE dbo.JobRecord SET error_occurred = 'True' WHERE epx_id =  " ("string"), w1303) -> (w1330:string)
                n552 = Concatenate Strings(w1339, w1340, w1330, w1327, w1329, w1310, w1299) -> (w1335:string)
                n553 = call-poly <vilib>:"DB Tools Execute Query.vi"("SQL query"=w1335, "connection reference"=w1334) -> ("error out"=w1326:errorcluster, "recordset reference"=w1341:T5)  [unwired: 6 in]
                n554 = call-poly <vilib>:"DB Tools Free Object.vi"("error in (no error)"=w1326, "recordset reference"=w1341) -> ("connection reference"=w1325:T4)  [unwired: 8 in, 1 out]
              }
            }
            n555 = call <vilib>:"DB Tools Close Connection.vi"("error in (no error)"=w1244, "connection reference"=w1245) -> ("error out"=w1252:errorcluster)  [unwired: 5 in]
            n556 = local write "error in (no error)"(w1252) -> ()
          }
        }
        n557 = case shown="False" "Stop" {
          selector: "Stop" -> [w39 w40]
          tunnel: [w39 w40] -> w34
          frame False {
          }
          frame True {
            n558 = invoke on="Indicator TAG" class="Str" method="Reinit To Default"() -> ()  [unwired: 3 in, 3 out]
            n559 = invoke on="Result: XML Header" class="Str" method="Reinit To Default"() -> ()  [unwired: 3 in, 3 out]
            n560 = invoke on="Control TAG" class="Str" method="Reinit To Default"() -> ()  [unwired: 3 in, 3 out]
            n561 = invoke on="Status" class="Str" method="Reinit To Default"() -> ()  [unwired: 3 in, 3 out]
            n562 = invoke on="Experiment VI" class="Str" method="Reinit To Default"() -> ()  [unwired: 3 in, 3 out]
            n563 = invoke on="Result: XML Footer" class="Str" method="Reinit To Default"() -> ()  [unwired: 3 in, 3 out]
            n564 = invoke on="Stop" class="Bool (strict)" method="Reinit To Default"() -> ()  [unwired: 3 in, 3 out]
            n565 = invoke on="Database" class="Str" method="Reinit To Default"() -> ()  [unwired: 3 in, 3 out]
          }
        }
        n566 = property on="Status" class="Str"("Text.Scroll Position"=inf) -> ()  [unwired: 2 in, 2 out]
      }
    }
  }
